vi "Wilt Prototype.vi"() -> ()   [LabVIEW 2009]
uses:
  Globals Wilt.vi
  Dryer.ctl
  Dryer Details.ctl
  Agilent Channel Definition.ctl
panel:
  out "Agilent Channels Array":T1[](array[typedef])
  out "Agilent Station Data Index Array":i32[][](array[numeric])
  out "Agilent Station Data Headers":string[][](array[string])
  in  "GUI Aisle 1A":T2[](array[typedef])=[{"Serial Number"="", "Cycle Count"=0.0, "Station Number"=0, "Dryer Details"={"Station"="", "Cycle Count"="", "Status"="", "Debug ASCII"="", "Note"="", "FILEMNAME"="", "Serial Number"="", "Total Time Drying"=""}, "Sample Record(t, Cycle Count, t-cum,L1, L2, V, Trmb, ASCII, Status) "=[], "Hist Record(Cycle Count, t-comp,L1max, L2max, Tmax) "=[], "Status Color"=0, "Boolean"=FALSE}, {"Serial Number"="", "Cycle Count"=0.0, "Station Number"=0, "Dryer Details"={"Station"="", "Cycle Count"="", "Status"="", "Debug ASCII"="", "Note"="", "FILEMNAME"="", "Serial Number"="", "Total Time Drying"=""}, "Sample Record(t, Cycle Count, t-cum,L1, L2, V, Trmb, ASCII, Status) "=[], "Hist Record(Cycle Count, t-comp,L1max, L2max, Tmax) "=[], "Status Color"=0, "Boolean"=FALSE}, {"Serial Number"="", "Cycle Count"=0.0, "Station Number"=0, "Dryer Details"={"Station"="", "Cycle Count"="", "Status"="", "Debug ASCII"="", "Note"="", "FILEMNAME"="", "Serial Number"="", "Total Time Drying"=""}, "Sample Record(t, Cycle Count, t-cum,L1, L2, V, Trmb, ASCII, Status) "=[], "Hist Record(Cycle Count, t-comp,L1max, L2max, Tmax) "=[], "Status Color"=0, "Boolean"=FALSE}, {"Serial Number"="", "Cycle Count"=0.0, "Station Number"=0, "Dryer Details"={"Station"="", "Cycle Count"="", "Status"="", "Debug ASCII"="", "Note"="", "FILEMNAME"="", "Serial Number"="", "Total Time Drying"=""}, "Sample Record(t, Cycle Count, t-cum,L1, L2, V, Trmb, ASCII, Status) "=[], "Hist Record(Cycle Count, t-comp,L1max, L2max, Tmax) "=[], "Status Color"=0, "Boolean"=FALSE}, {"Serial Number"="", "Cycle Count"=0.0, "Station Number"=0, "Dryer Details"={"Station"="", "Cycle Count"="", "Status"="", "Debug ASCII"="", "Note"="", "FILEMNAME"="", "Serial Number"="", "Total Time Drying"=""}, "Sample Record(t, Cycle Count, t-cum,L1, L2, V, Trmb, ASCII, Status) "=[], "Hist Record(Cycle Count, t-comp,L1max, L2max, Tmax) "=[], "Status Color"=0, "Boolean"=FALSE}, {"Serial Number"="", "Cycle Count"=0.0, "Station Number"=0, "Dryer Details"={"Station"="", "Cycle Count"="", "Status"="", "Debug ASCII"="", "Note"="", "FILEMNAME"="", "Serial Number"="", "Total Time Drying"=""}, "Sample Record(t, Cycle Count, t-cum,L1, L2, V, Trmb, ASCII, Status) "=[], "Hist Record(Cycle Count, t-comp,L1max, L2max, Tmax) "=[], "Status Color"=0, "Boolean"=FALSE}, {"Serial Number"="", "Cycle Count"=0.0, "Station Number"=0, "Dryer Details"={"Station"="", "Cycle Count"="", "Status"="", "Debug ASCII"="", "Note"="", "FILEMNAME"="", "Serial Number"="", "Total Time Drying"=""}, "Sample Record(t, Cycle Count, t-cum,L1, L2, V, Trmb, ASCII, Status) "=[], "Hist Record(Cycle Count, t-comp,L1max, L2max, Tmax) "=[], "Status Color"=0, "Boolean"=FALSE}, {"Serial Number"="", "Cycle Count"=0.0, "Station Number"=0, "Dryer Details"={"Station"="", "Cycle Count"="", "Status"="", "Debug ASCII"="", "Note"="", "FILEMNAME"="", "Serial Number"="", "Total Time Drying"=""}, "Sample Record(t, Cycle Count, t-cum,L1, L2, V, Trmb, ASCII, Status) "=[], "Hist Record(Cycle Count, t-comp,L1max, L2max, Tmax) "=[], "Status Color"=0, "Boolean"=TRUE}] {"Station Number" format="%02.0f"; "Cycle Count" format="%0#4_4g"}
  in  "GUI Aisle 1":T2[](array[typedef])=[{"Serial Number"="", "Cycle Count"=0.0, "Station Number"=0, "Dryer Details"={"Station"="", "Cycle Count"="", "Status"="", "Debug ASCII"="", "Note"="", "FILEMNAME"="", "Serial Number"="", "Total Time Drying"=""}, "Sample Record(t, Cycle Count, t-cum,L1, L2, V, Trmb, ASCII, Status) "=[], "Hist Record(Cycle Count, t-comp,L1max, L2max, Tmax) "=[], "Status Color"=0, "Boolean"=FALSE}, {"Serial Number"="", "Cycle Count"=0.0, "Station Number"=0, "Dryer Details"={"Station"="", "Cycle Count"="", "Status"="", "Debug ASCII"="", "Note"="", "FILEMNAME"="", "Serial Number"="", "Total Time Drying"=""}, "Sample Record(t, Cycle Count, t-cum,L1, L2, V, Trmb, ASCII, Status) "=[], "Hist Record(Cycle Count, t-comp,L1max, L2max, Tmax) "=[], "Status Color"=0, "Boolean"=FALSE}, {"Serial Number"="", "Cycle Count"=0.0, "Station Number"=0, "Dryer Details"={"Station"="", "Cycle Count"="", "Status"="", "Debug ASCII"="", "Note"="", "FILEMNAME"="", "Serial Number"="", "Total Time Drying"=""}, "Sample Record(t, Cycle Count, t-cum,L1, L2, V, Trmb, ASCII, Status) "=[], "Hist Record(Cycle Count, t-comp,L1max, L2max, Tmax) "=[], "Status Color"=0, "Boolean"=FALSE}, {"Serial Number"="", "Cycle Count"=0.0, "Station Number"=0, "Dryer Details"={"Station"="", "Cycle Count"="", "Status"="", "Debug ASCII"="", "Note"="", "FILEMNAME"="", "Serial Number"="", "Total Time Drying"=""}, "Sample Record(t, Cycle Count, t-cum,L1, L2, V, Trmb, ASCII, Status) "=[], "Hist Record(Cycle Count, t-comp,L1max, L2max, Tmax) "=[], "Status Color"=0, "Boolean"=FALSE}, {"Serial Number"="", "Cycle Count"=0.0, "Station Number"=0, "Dryer Details"={"Station"="", "Cycle Count"="", "Status"="", "Debug ASCII"="", "Note"="", "FILEMNAME"="", "Serial Number"="", "Total Time Drying"=""}, "Sample Record(t, Cycle Count, t-cum,L1, L2, V, Trmb, ASCII, Status) "=[], "Hist Record(Cycle Count, t-comp,L1max, L2max, Tmax) "=[], "Status Color"=0, "Boolean"=FALSE}, {"Serial Number"="", "Cycle Count"=0.0, "Station Number"=0, "Dryer Details"={"Station"="", "Cycle Count"="", "Status"="", "Debug ASCII"="", "Note"="", "FILEMNAME"="", "Serial Number"="", "Total Time Drying"=""}, "Sample Record(t, Cycle Count, t-cum,L1, L2, V, Trmb, ASCII, Status) "=[], "Hist Record(Cycle Count, t-comp,L1max, L2max, Tmax) "=[], "Status Color"=0, "Boolean"=FALSE}, {"Serial Number"="", "Cycle Count"=0.0, "Station Number"=0, "Dryer Details"={"Station"="", "Cycle Count"="", "Status"="", "Debug ASCII"="", "Note"="", "FILEMNAME"="", "Serial Number"="", "Total Time Drying"=""}, "Sample Record(t, Cycle Count, t-cum,L1, L2, V, Trmb, ASCII, Status) "=[], "Hist Record(Cycle Count, t-comp,L1max, L2max, Tmax) "=[], "Status Color"=0, "Boolean"=FALSE}, {"Serial Number"="", "Cycle Count"=0.0, "Station Number"=0, "Dryer Details"={"Station"="", "Cycle Count"="", "Status"="", "Debug ASCII"="", "Note"="", "FILEMNAME"="", "Serial Number"="", "Total Time Drying"=""}, "Sample Record(t, Cycle Count, t-cum,L1, L2, V, Trmb, ASCII, Status) "=[], "Hist Record(Cycle Count, t-comp,L1max, L2max, Tmax) "=[], "Status Color"=0, "Boolean"=FALSE}, {"Serial Number"="", "Cycle Count"=0.0, "Station Number"=0, "Dryer Details"={"Station"="", "Cycle Count"="", "Status"="", "Debug ASCII"="", "Note"="", "FILEMNAME"="", "Serial Number"="", "Total Time Drying"=""}, "Sample Record(t, Cycle Count, t-cum,L1, L2, V, Trmb, ASCII, Status) "=[], "Hist Record(Cycle Count, t-comp,L1max, L2max, Tmax) "=[], "Status Color"=0, "Boolean"=FALSE}, {"Serial Number"="", "Cycle Count"=0.0, "Station Number"=0, "Dryer Details"={"Station"="", "Cycle Count"="", "Status"="", "Debug ASCII"="", "Note"="", "FILEMNAME"="", "Serial Number"="", "Total Time Drying"=""}, "Sample Record(t, Cycle Count, t-cum,L1, L2, V, Trmb, ASCII, Status) "=[], "Hist Record(Cycle Count, t-comp,L1max, L2max, Tmax) "=[], "Status Color"=0, "Boolean"=FALSE}, {"Serial Number"="", "Cycle Count"=0.0, "Station Number"=0, "Dryer Details"={"Station"="", "Cycle Count"="", "Status"="", "Debug ASCII"="", "Note"="", "FILEMNAME"="", "Serial Number"="", "Total Time Drying"=""}, "Sample Record(t, Cycle Count, t-cum,L1, L2, V, Trmb, ASCII, Status) "=[], "Hist Record(Cycle Count, t-comp,L1max, L2max, Tmax) "=[], "Status Color"=0, "Boolean"=FALSE}, {"Serial Number"="", "Cycle Count"=0.0, "Station Number"=0, "Dryer Details"={"Station"="", "Cycle Count"="", "Status"="", "Debug ASCII"="", "Note"="", "FILEMNAME"="", "Serial Number"="", "Total Time Drying"=""}, "Sample Record(t, Cycle Count, t-cum,L1, L2, V, Trmb, ASCII, Status) "=[], "Hist Record(Cycle Count, t-comp,L1max, L2max, Tmax) "=[], "Status Color"=0, "Boolean"=TRUE}] {"Station Number" format="%02.0f"; "Cycle Count" format="%0#4_4g"}
  in  "GUI Aisle 2":T2[](array[typedef])=[{"Serial Number"="", "Cycle Count"=0.0, "Station Number"=0, "Dryer Details"={"Station"="", "Cycle Count"="", "Status"="", "Debug ASCII"="", "Note"="", "FILEMNAME"="", "Serial Number"="", "Total Time Drying"=""}, "Sample Record(t, Cycle Count, t-cum,L1, L2, V, Trmb, ASCII, Status) "=[], "Hist Record(Cycle Count, t-comp,L1max, L2max, Tmax) "=[], "Status Color"=0, "Boolean"=FALSE}, {"Serial Number"="", "Cycle Count"=0.0, "Station Number"=0, "Dryer Details"={"Station"="", "Cycle Count"="", "Status"="", "Debug ASCII"="", "Note"="", "FILEMNAME"="", "Serial Number"="", "Total Time Drying"=""}, "Sample Record(t, Cycle Count, t-cum,L1, L2, V, Trmb, ASCII, Status) "=[], "Hist Record(Cycle Count, t-comp,L1max, L2max, Tmax) "=[], "Status Color"=0, "Boolean"=FALSE}, {"Serial Number"="", "Cycle Count"=0.0, "Station Number"=0, "Dryer Details"={"Station"="", "Cycle Count"="", "Status"="", "Debug ASCII"="", "Note"="", "FILEMNAME"="", "Serial Number"="", "Total Time Drying"=""}, "Sample Record(t, Cycle Count, t-cum,L1, L2, V, Trmb, ASCII, Status) "=[], "Hist Record(Cycle Count, t-comp,L1max, L2max, Tmax) "=[], "Status Color"=0, "Boolean"=FALSE}, {"Serial Number"="", "Cycle Count"=0.0, "Station Number"=0, "Dryer Details"={"Station"="", "Cycle Count"="", "Status"="", "Debug ASCII"="", "Note"="", "FILEMNAME"="", "Serial Number"="", "Total Time Drying"=""}, "Sample Record(t, Cycle Count, t-cum,L1, L2, V, Trmb, ASCII, Status) "=[], "Hist Record(Cycle Count, t-comp,L1max, L2max, Tmax) "=[], "Status Color"=0, "Boolean"=FALSE}, {"Serial Number"="", "Cycle Count"=0.0, "Station Number"=0, "Dryer Details"={"Station"="", "Cycle Count"="", "Status"="", "Debug ASCII"="", "Note"="", "FILEMNAME"="", "Serial Number"="", "Total Time Drying"=""}, "Sample Record(t, Cycle Count, t-cum,L1, L2, V, Trmb, ASCII, Status) "=[], "Hist Record(Cycle Count, t-comp,L1max, L2max, Tmax) "=[], "Status Color"=0, "Boolean"=FALSE}, {"Serial Number"="", "Cycle Count"=0.0, "Station Number"=0, "Dryer Details"={"Station"="", "Cycle Count"="", "Status"="", "Debug ASCII"="", "Note"="", "FILEMNAME"="", "Serial Number"="", "Total Time Drying"=""}, "Sample Record(t, Cycle Count, t-cum,L1, L2, V, Trmb, ASCII, Status) "=[], "Hist Record(Cycle Count, t-comp,L1max, L2max, Tmax) "=[], "Status Color"=0, "Boolean"=FALSE}, {"Serial Number"="", "Cycle Count"=0.0, "Station Number"=0, "Dryer Details"={"Station"="", "Cycle Count"="", "Status"="", "Debug ASCII"="", "Note"="", "FILEMNAME"="", "Serial Number"="", "Total Time Drying"=""}, "Sample Record(t, Cycle Count, t-cum,L1, L2, V, Trmb, ASCII, Status) "=[], "Hist Record(Cycle Count, t-comp,L1max, L2max, Tmax) "=[], "Status Color"=0, "Boolean"=FALSE}, {"Serial Number"="", "Cycle Count"=0.0, "Station Number"=0, "Dryer Details"={"Station"="", "Cycle Count"="", "Status"="", "Debug ASCII"="", "Note"="", "FILEMNAME"="", "Serial Number"="", "Total Time Drying"=""}, "Sample Record(t, Cycle Count, t-cum,L1, L2, V, Trmb, ASCII, Status) "=[], "Hist Record(Cycle Count, t-comp,L1max, L2max, Tmax) "=[], "Status Color"=0, "Boolean"=FALSE}, {"Serial Number"="", "Cycle Count"=0.0, "Station Number"=0, "Dryer Details"={"Station"="", "Cycle Count"="", "Status"="", "Debug ASCII"="", "Note"="", "FILEMNAME"="", "Serial Number"="", "Total Time Drying"=""}, "Sample Record(t, Cycle Count, t-cum,L1, L2, V, Trmb, ASCII, Status) "=[], "Hist Record(Cycle Count, t-comp,L1max, L2max, Tmax) "=[], "Status Color"=0, "Boolean"=FALSE}, {"Serial Number"="", "Cycle Count"=0.0, "Station Number"=0, "Dryer Details"={"Station"="", "Cycle Count"="", "Status"="", "Debug ASCII"="", "Note"="", "FILEMNAME"="", "Serial Number"="", "Total Time Drying"=""}, "Sample Record(t, Cycle Count, t-cum,L1, L2, V, Trmb, ASCII, Status) "=[], "Hist Record(Cycle Count, t-comp,L1max, L2max, Tmax) "=[], "Status Color"=0, "Boolean"=FALSE}, {"Serial Number"="", "Cycle Count"=0.0, "Station Number"=0, "Dryer Details"={"Station"="", "Cycle Count"="", "Status"="", "Debug ASCII"="", "Note"="", "FILEMNAME"="", "Serial Number"="", "Total Time Drying"=""}, "Sample Record(t, Cycle Count, t-cum,L1, L2, V, Trmb, ASCII, Status) "=[], "Hist Record(Cycle Count, t-comp,L1max, L2max, Tmax) "=[], "Status Color"=0, "Boolean"=FALSE}, {"Serial Number"="", "Cycle Count"=0.0, "Station Number"=0, "Dryer Details"={"Station"="", "Cycle Count"="", "Status"="", "Debug ASCII"="", "Note"="", "FILEMNAME"="", "Serial Number"="", "Total Time Drying"=""}, "Sample Record(t, Cycle Count, t-cum,L1, L2, V, Trmb, ASCII, Status) "=[], "Hist Record(Cycle Count, t-comp,L1max, L2max, Tmax) "=[], "Status Color"=0, "Boolean"=TRUE}] {"Station Number" format="%02.0f"; "Cycle Count" format="%0#4_4g"}
  in  "GUI Aisle 3":T2[](array[typedef])=[{"Serial Number"="", "Cycle Count"=0.0, "Station Number"=0, "Dryer Details"={"Station"="", "Cycle Count"="", "Status"="", "Debug ASCII"="", "Note"="", "FILEMNAME"="", "Serial Number"="", "Total Time Drying"=""}, "Sample Record(t, Cycle Count, t-cum,L1, L2, V, Trmb, ASCII, Status) "=[], "Hist Record(Cycle Count, t-comp,L1max, L2max, Tmax) "=[], "Status Color"=0, "Boolean"=FALSE}, {"Serial Number"="", "Cycle Count"=0.0, "Station Number"=0, "Dryer Details"={"Station"="", "Cycle Count"="", "Status"="", "Debug ASCII"="", "Note"="", "FILEMNAME"="", "Serial Number"="", "Total Time Drying"=""}, "Sample Record(t, Cycle Count, t-cum,L1, L2, V, Trmb, ASCII, Status) "=[], "Hist Record(Cycle Count, t-comp,L1max, L2max, Tmax) "=[], "Status Color"=0, "Boolean"=FALSE}, {"Serial Number"="", "Cycle Count"=0.0, "Station Number"=0, "Dryer Details"={"Station"="", "Cycle Count"="", "Status"="", "Debug ASCII"="", "Note"="", "FILEMNAME"="", "Serial Number"="", "Total Time Drying"=""}, "Sample Record(t, Cycle Count, t-cum,L1, L2, V, Trmb, ASCII, Status) "=[], "Hist Record(Cycle Count, t-comp,L1max, L2max, Tmax) "=[], "Status Color"=0, "Boolean"=FALSE}, {"Serial Number"="", "Cycle Count"=0.0, "Station Number"=0, "Dryer Details"={"Station"="", "Cycle Count"="", "Status"="", "Debug ASCII"="", "Note"="", "FILEMNAME"="", "Serial Number"="", "Total Time Drying"=""}, "Sample Record(t, Cycle Count, t-cum,L1, L2, V, Trmb, ASCII, Status) "=[], "Hist Record(Cycle Count, t-comp,L1max, L2max, Tmax) "=[], "Status Color"=0, "Boolean"=FALSE}, {"Serial Number"="", "Cycle Count"=0.0, "Station Number"=0, "Dryer Details"={"Station"="", "Cycle Count"="", "Status"="", "Debug ASCII"="", "Note"="", "FILEMNAME"="", "Serial Number"="", "Total Time Drying"=""}, "Sample Record(t, Cycle Count, t-cum,L1, L2, V, Trmb, ASCII, Status) "=[], "Hist Record(Cycle Count, t-comp,L1max, L2max, Tmax) "=[], "Status Color"=0, "Boolean"=FALSE}, {"Serial Number"="", "Cycle Count"=0.0, "Station Number"=0, "Dryer Details"={"Station"="", "Cycle Count"="", "Status"="", "Debug ASCII"="", "Note"="", "FILEMNAME"="", "Serial Number"="", "Total Time Drying"=""}, "Sample Record(t, Cycle Count, t-cum,L1, L2, V, Trmb, ASCII, Status) "=[], "Hist Record(Cycle Count, t-comp,L1max, L2max, Tmax) "=[], "Status Color"=0, "Boolean"=FALSE}, {"Serial Number"="", "Cycle Count"=0.0, "Station Number"=0, "Dryer Details"={"Station"="", "Cycle Count"="", "Status"="", "Debug ASCII"="", "Note"="", "FILEMNAME"="", "Serial Number"="", "Total Time Drying"=""}, "Sample Record(t, Cycle Count, t-cum,L1, L2, V, Trmb, ASCII, Status) "=[], "Hist Record(Cycle Count, t-comp,L1max, L2max, Tmax) "=[], "Status Color"=0, "Boolean"=FALSE}, {"Serial Number"="", "Cycle Count"=0.0, "Station Number"=0, "Dryer Details"={"Station"="", "Cycle Count"="", "Status"="", "Debug ASCII"="", "Note"="", "FILEMNAME"="", "Serial Number"="", "Total Time Drying"=""}, "Sample Record(t, Cycle Count, t-cum,L1, L2, V, Trmb, ASCII, Status) "=[], "Hist Record(Cycle Count, t-comp,L1max, L2max, Tmax) "=[], "Status Color"=0, "Boolean"=FALSE}, {"Serial Number"="", "Cycle Count"=0.0, "Station Number"=0, "Dryer Details"={"Station"="", "Cycle Count"="", "Status"="", "Debug ASCII"="", "Note"="", "FILEMNAME"="", "Serial Number"="", "Total Time Drying"=""}, "Sample Record(t, Cycle Count, t-cum,L1, L2, V, Trmb, ASCII, Status) "=[], "Hist Record(Cycle Count, t-comp,L1max, L2max, Tmax) "=[], "Status Color"=0, "Boolean"=FALSE}, {"Serial Number"="", "Cycle Count"=0.0, "Station Number"=0, "Dryer Details"={"Station"="", "Cycle Count"="", "Status"="", "Debug ASCII"="", "Note"="", "FILEMNAME"="", "Serial Number"="", "Total Time Drying"=""}, "Sample Record(t, Cycle Count, t-cum,L1, L2, V, Trmb, ASCII, Status) "=[], "Hist Record(Cycle Count, t-comp,L1max, L2max, Tmax) "=[], "Status Color"=0, "Boolean"=FALSE}, {"Serial Number"="", "Cycle Count"=0.0, "Station Number"=0, "Dryer Details"={"Station"="", "Cycle Count"="", "Status"="", "Debug ASCII"="", "Note"="", "FILEMNAME"="", "Serial Number"="", "Total Time Drying"=""}, "Sample Record(t, Cycle Count, t-cum,L1, L2, V, Trmb, ASCII, Status) "=[], "Hist Record(Cycle Count, t-comp,L1max, L2max, Tmax) "=[], "Status Color"=0, "Boolean"=FALSE}, {"Serial Number"="", "Cycle Count"=0.0, "Station Number"=0, "Dryer Details"={"Station"="", "Cycle Count"="", "Status"="", "Debug ASCII"="", "Note"="", "FILEMNAME"="", "Serial Number"="", "Total Time Drying"=""}, "Sample Record(t, Cycle Count, t-cum,L1, L2, V, Trmb, ASCII, Status) "=[], "Hist Record(Cycle Count, t-comp,L1max, L2max, Tmax) "=[], "Status Color"=0, "Boolean"=TRUE}] {"Station Number" format="%02.0f"; "Cycle Count" format="%0#4_4g"}
  in  "GUI Aisle 4":T2[](array[typedef])=[{"Serial Number"="", "Cycle Count"=0.0, "Station Number"=0, "Dryer Details"={"Station"="", "Cycle Count"="", "Status"="", "Debug ASCII"="", "Note"="", "FILEMNAME"="", "Serial Number"="", "Total Time Drying"=""}, "Sample Record(t, Cycle Count, t-cum,L1, L2, V, Trmb, ASCII, Status) "=[], "Hist Record(Cycle Count, t-comp,L1max, L2max, Tmax) "=[], "Status Color"=0, "Boolean"=FALSE}, {"Serial Number"="", "Cycle Count"=0.0, "Station Number"=0, "Dryer Details"={"Station"="", "Cycle Count"="", "Status"="", "Debug ASCII"="", "Note"="", "FILEMNAME"="", "Serial Number"="", "Total Time Drying"=""}, "Sample Record(t, Cycle Count, t-cum,L1, L2, V, Trmb, ASCII, Status) "=[], "Hist Record(Cycle Count, t-comp,L1max, L2max, Tmax) "=[], "Status Color"=0, "Boolean"=FALSE}, {"Serial Number"="", "Cycle Count"=0.0, "Station Number"=0, "Dryer Details"={"Station"="", "Cycle Count"="", "Status"="", "Debug ASCII"="", "Note"="", "FILEMNAME"="", "Serial Number"="", "Total Time Drying"=""}, "Sample Record(t, Cycle Count, t-cum,L1, L2, V, Trmb, ASCII, Status) "=[], "Hist Record(Cycle Count, t-comp,L1max, L2max, Tmax) "=[], "Status Color"=0, "Boolean"=FALSE}, {"Serial Number"="", "Cycle Count"=0.0, "Station Number"=0, "Dryer Details"={"Station"="", "Cycle Count"="", "Status"="", "Debug ASCII"="", "Note"="", "FILEMNAME"="", "Serial Number"="", "Total Time Drying"=""}, "Sample Record(t, Cycle Count, t-cum,L1, L2, V, Trmb, ASCII, Status) "=[], "Hist Record(Cycle Count, t-comp,L1max, L2max, Tmax) "=[], "Status Color"=0, "Boolean"=FALSE}, {"Serial Number"="", "Cycle Count"=0.0, "Station Number"=0, "Dryer Details"={"Station"="", "Cycle Count"="", "Status"="", "Debug ASCII"="", "Note"="", "FILEMNAME"="", "Serial Number"="", "Total Time Drying"=""}, "Sample Record(t, Cycle Count, t-cum,L1, L2, V, Trmb, ASCII, Status) "=[], "Hist Record(Cycle Count, t-comp,L1max, L2max, Tmax) "=[], "Status Color"=0, "Boolean"=FALSE}, {"Serial Number"="", "Cycle Count"=0.0, "Station Number"=0, "Dryer Details"={"Station"="", "Cycle Count"="", "Status"="", "Debug ASCII"="", "Note"="", "FILEMNAME"="", "Serial Number"="", "Total Time Drying"=""}, "Sample Record(t, Cycle Count, t-cum,L1, L2, V, Trmb, ASCII, Status) "=[], "Hist Record(Cycle Count, t-comp,L1max, L2max, Tmax) "=[], "Status Color"=0, "Boolean"=FALSE}, {"Serial Number"="", "Cycle Count"=0.0, "Station Number"=0, "Dryer Details"={"Station"="", "Cycle Count"="", "Status"="", "Debug ASCII"="", "Note"="", "FILEMNAME"="", "Serial Number"="", "Total Time Drying"=""}, "Sample Record(t, Cycle Count, t-cum,L1, L2, V, Trmb, ASCII, Status) "=[], "Hist Record(Cycle Count, t-comp,L1max, L2max, Tmax) "=[], "Status Color"=0, "Boolean"=FALSE}, {"Serial Number"="", "Cycle Count"=0.0, "Station Number"=0, "Dryer Details"={"Station"="", "Cycle Count"="", "Status"="", "Debug ASCII"="", "Note"="", "FILEMNAME"="", "Serial Number"="", "Total Time Drying"=""}, "Sample Record(t, Cycle Count, t-cum,L1, L2, V, Trmb, ASCII, Status) "=[], "Hist Record(Cycle Count, t-comp,L1max, L2max, Tmax) "=[], "Status Color"=0, "Boolean"=FALSE}, {"Serial Number"="", "Cycle Count"=0.0, "Station Number"=0, "Dryer Details"={"Station"="", "Cycle Count"="", "Status"="", "Debug ASCII"="", "Note"="", "FILEMNAME"="", "Serial Number"="", "Total Time Drying"=""}, "Sample Record(t, Cycle Count, t-cum,L1, L2, V, Trmb, ASCII, Status) "=[], "Hist Record(Cycle Count, t-comp,L1max, L2max, Tmax) "=[], "Status Color"=0, "Boolean"=FALSE}, {"Serial Number"="", "Cycle Count"=0.0, "Station Number"=0, "Dryer Details"={"Station"="", "Cycle Count"="", "Status"="", "Debug ASCII"="", "Note"="", "FILEMNAME"="", "Serial Number"="", "Total Time Drying"=""}, "Sample Record(t, Cycle Count, t-cum,L1, L2, V, Trmb, ASCII, Status) "=[], "Hist Record(Cycle Count, t-comp,L1max, L2max, Tmax) "=[], "Status Color"=0, "Boolean"=FALSE}, {"Serial Number"="", "Cycle Count"=0.0, "Station Number"=0, "Dryer Details"={"Station"="", "Cycle Count"="", "Status"="", "Debug ASCII"="", "Note"="", "FILEMNAME"="", "Serial Number"="", "Total Time Drying"=""}, "Sample Record(t, Cycle Count, t-cum,L1, L2, V, Trmb, ASCII, Status) "=[], "Hist Record(Cycle Count, t-comp,L1max, L2max, Tmax) "=[], "Status Color"=0, "Boolean"=FALSE}, {"Serial Number"="", "Cycle Count"=0.0, "Station Number"=0, "Dryer Details"={"Station"="", "Cycle Count"="", "Status"="", "Debug ASCII"="", "Note"="", "FILEMNAME"="", "Serial Number"="", "Total Time Drying"=""}, "Sample Record(t, Cycle Count, t-cum,L1, L2, V, Trmb, ASCII, Status) "=[], "Hist Record(Cycle Count, t-comp,L1max, L2max, Tmax) "=[], "Status Color"=0, "Boolean"=TRUE}] {"Station Number" format="%02.0f"; "Cycle Count" format="%0#4_4g"}
  out "Elapsed Time (sec)":dbl format="%.2f"
  in  "Tab Control":enum32{"Config Variables", "Page 2", "Page 3"}(tab)
  in  "DAQ Delay":i32=1000
  out "All Com Array":i32[](array[numeric])=[100, 2, 3, 4, 5, 6, 7, 8, 9, 10, 11, 12, 13, 14, 15, 16, 17, 18, 19, 20, 21, 22, 23, 24, 25, 26, 27, 28, 29, 30, 31, 32, 33, 34, 35, 36, 37, 38, 39, 40, 41, 42, 43, 44, 45, 46, 47, 48, 49, 50, 51, 52, 53, 54, 55, 56]
  out "Init Complete":bool=TRUE
  out "Test Complete":bool
  in  "Simulation":bool
  in  "Data File Directory":path
  in  "Dryer To Save":T2 {"Station Number" format="%02.0f"; "Cycle Count" format="%0#4_4g"}
  out "Current Serial Output Array":string[](array[string])
  out "Agilent Refs":refnum<visa-resource-name>[](array[refnum])=["AGILENT1", "AGILENT2", "AGILENT3", "AGILENT4", "AGILENT5"]
  out "Agilent Refs Var":refnum<visa-resource-name>[](array[refnum])=["AGILENT1", "AGILENT2", "AGILENT3", "AGILENT4", "AGILENT5"]
  out "Current Agilent Data":dbl[][](array[numeric])
  out "Gathering Data Latch":bool=TRUE
  out "Current Status Array":cluster{"Color":u32, "Status":string}[](array[cluster])
  in  "Stop Test":bool
  in  "Fault":u32(colorbox)=16711680
  in  "Stopped":u32(colorbox)=16776960
  in  "Running":u32(colorbox)=6618880
  in  "No Com":u32(colorbox)
  # "WILT DRYER Test"
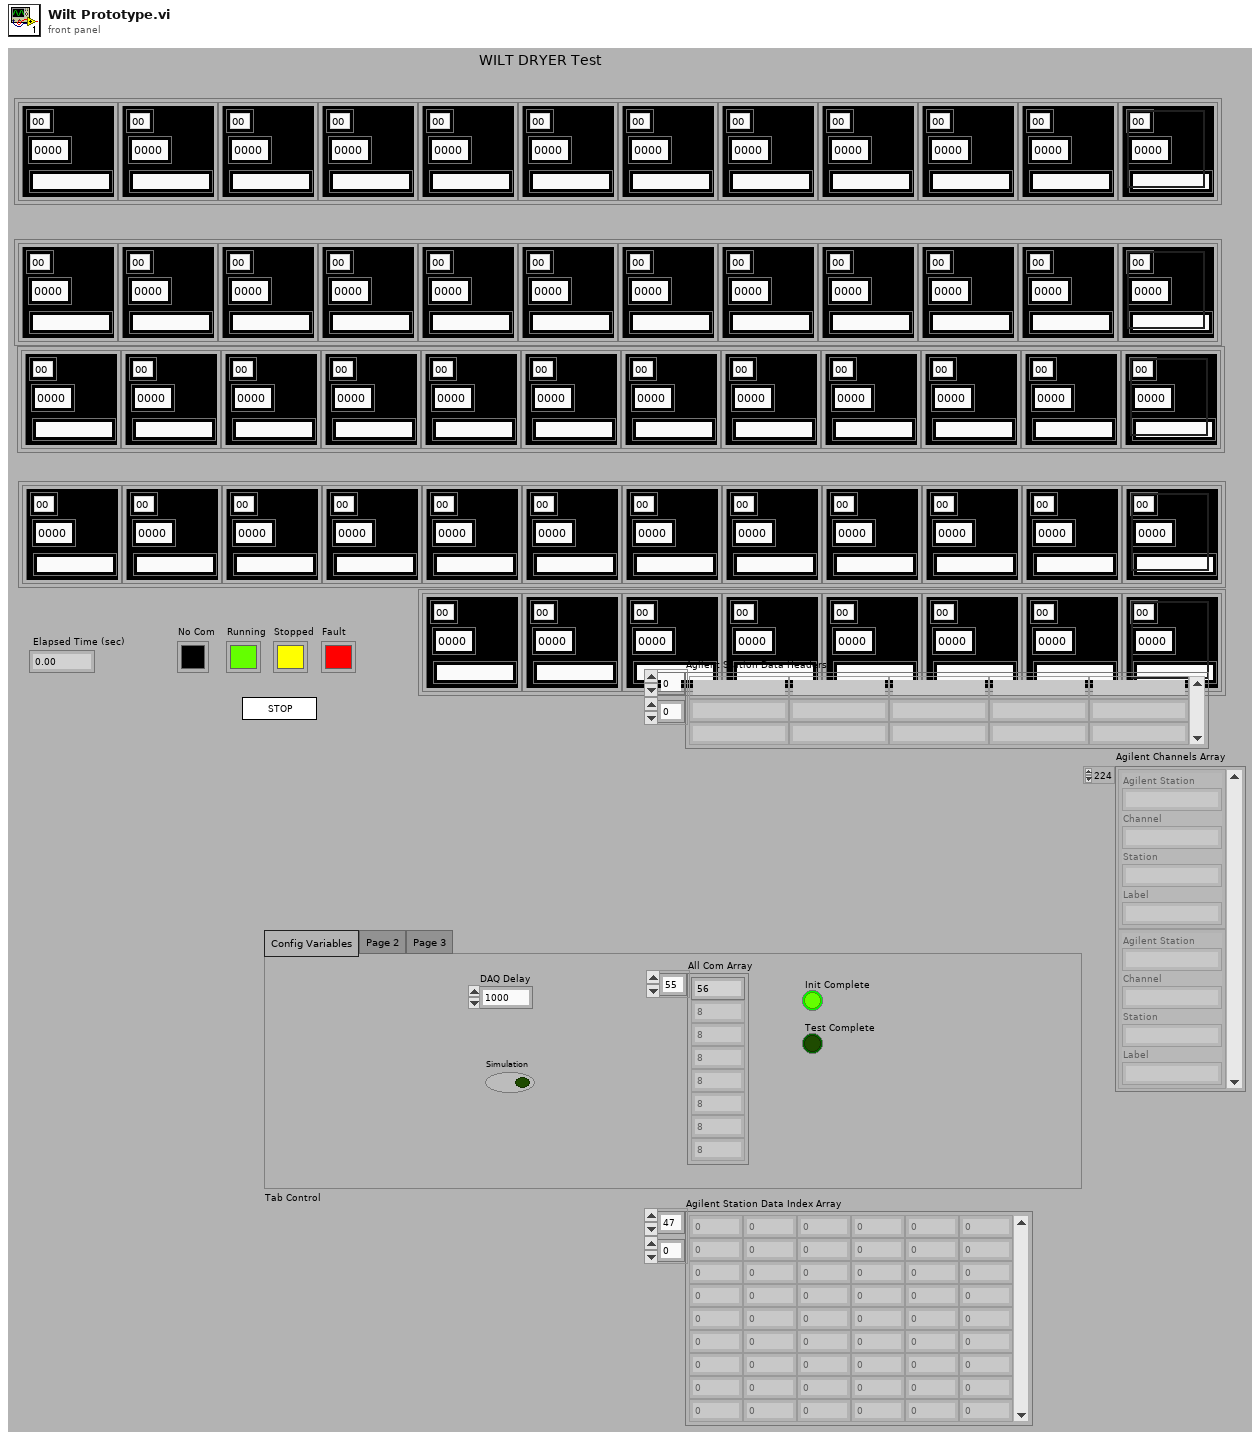
[diagram p1: front panel]
types:
  T1 = typedef "Agilent Channel Definition.ctl" = cluster{"Channel":string, "Station":string, "Label":string, "Agilent Station":string}
  T2 = typedef "Dryer.ctl" = cluster{"Serial Number":string, "Cycle Count":dbl, "Station Number":u8, "Dryer Details":T3, "Sample Record(t, Cycle Count, t-cum,L1, L2, V, Trmb, ASCII, Status) ":string[][], "Hist Record(Cycle Count, t-comp,L1max, L2max, Tmax) ":string[][], "Status Color":u32, "Boolean":bool}
  T3 = typedef "Dryer Details.ctl" = cluster{"Station":string, "Cycle Count":string, "Status":string, "Debug ASCII":string, "Note":string, "FILEMNAME":string, "Serial Number":string, "Total Time Drying":string}
  T4 = enum32{"invalid app kind", "Development System", "Run Time System", "Student Edition", "Embedded LabVIEW", "Evaluation", "Custom"}
  T5 = enum16{"Init Station Number", "Update Detail Data", "Update Status"}
  T6 = enum32{"Invalid", "Standard", "Closed", "Hidden", "Minimized", "Maximized"}
  T7 = cluster{"Core":cluster{"Current VI Reference":refnum<vi>, "Close Panel on Exit?":bool}, "UI Refs":refnum<vi>[], "Agilent Refs":refnum<visa-resource-name>[], "GUI Aisle 4":T2[], "GUI Aisle 3":T2[], "GUI Aisle 2":T2[], "GUI Aisle 1A":T2[], "GUI Aisle 1":T2[]}
  T8 = cluster{"Current VI Reference":refnum<vi>, "Close Panel on Exit?":bool}
  T9 = enum16{"Init Com Port", "SendCMD", "ReadPort", "Close Port", "Simulate Diag Data", "Simulate Dryer"}
  T10 = cluster{"GUI Aisle 1":T2[], "GUI Aisle 1A":T2[], "GUI Aisle 2":T2[], "GUI Aisle 3":T2[], "GUI Aisle 4":T2[], "Dryer To Save":T2}
  T11 = cluster{"Agilent Refs Var":refnum<visa-resource-name>[], "All Com Array":i32[], "Elapsed Time (sec)":dbl}
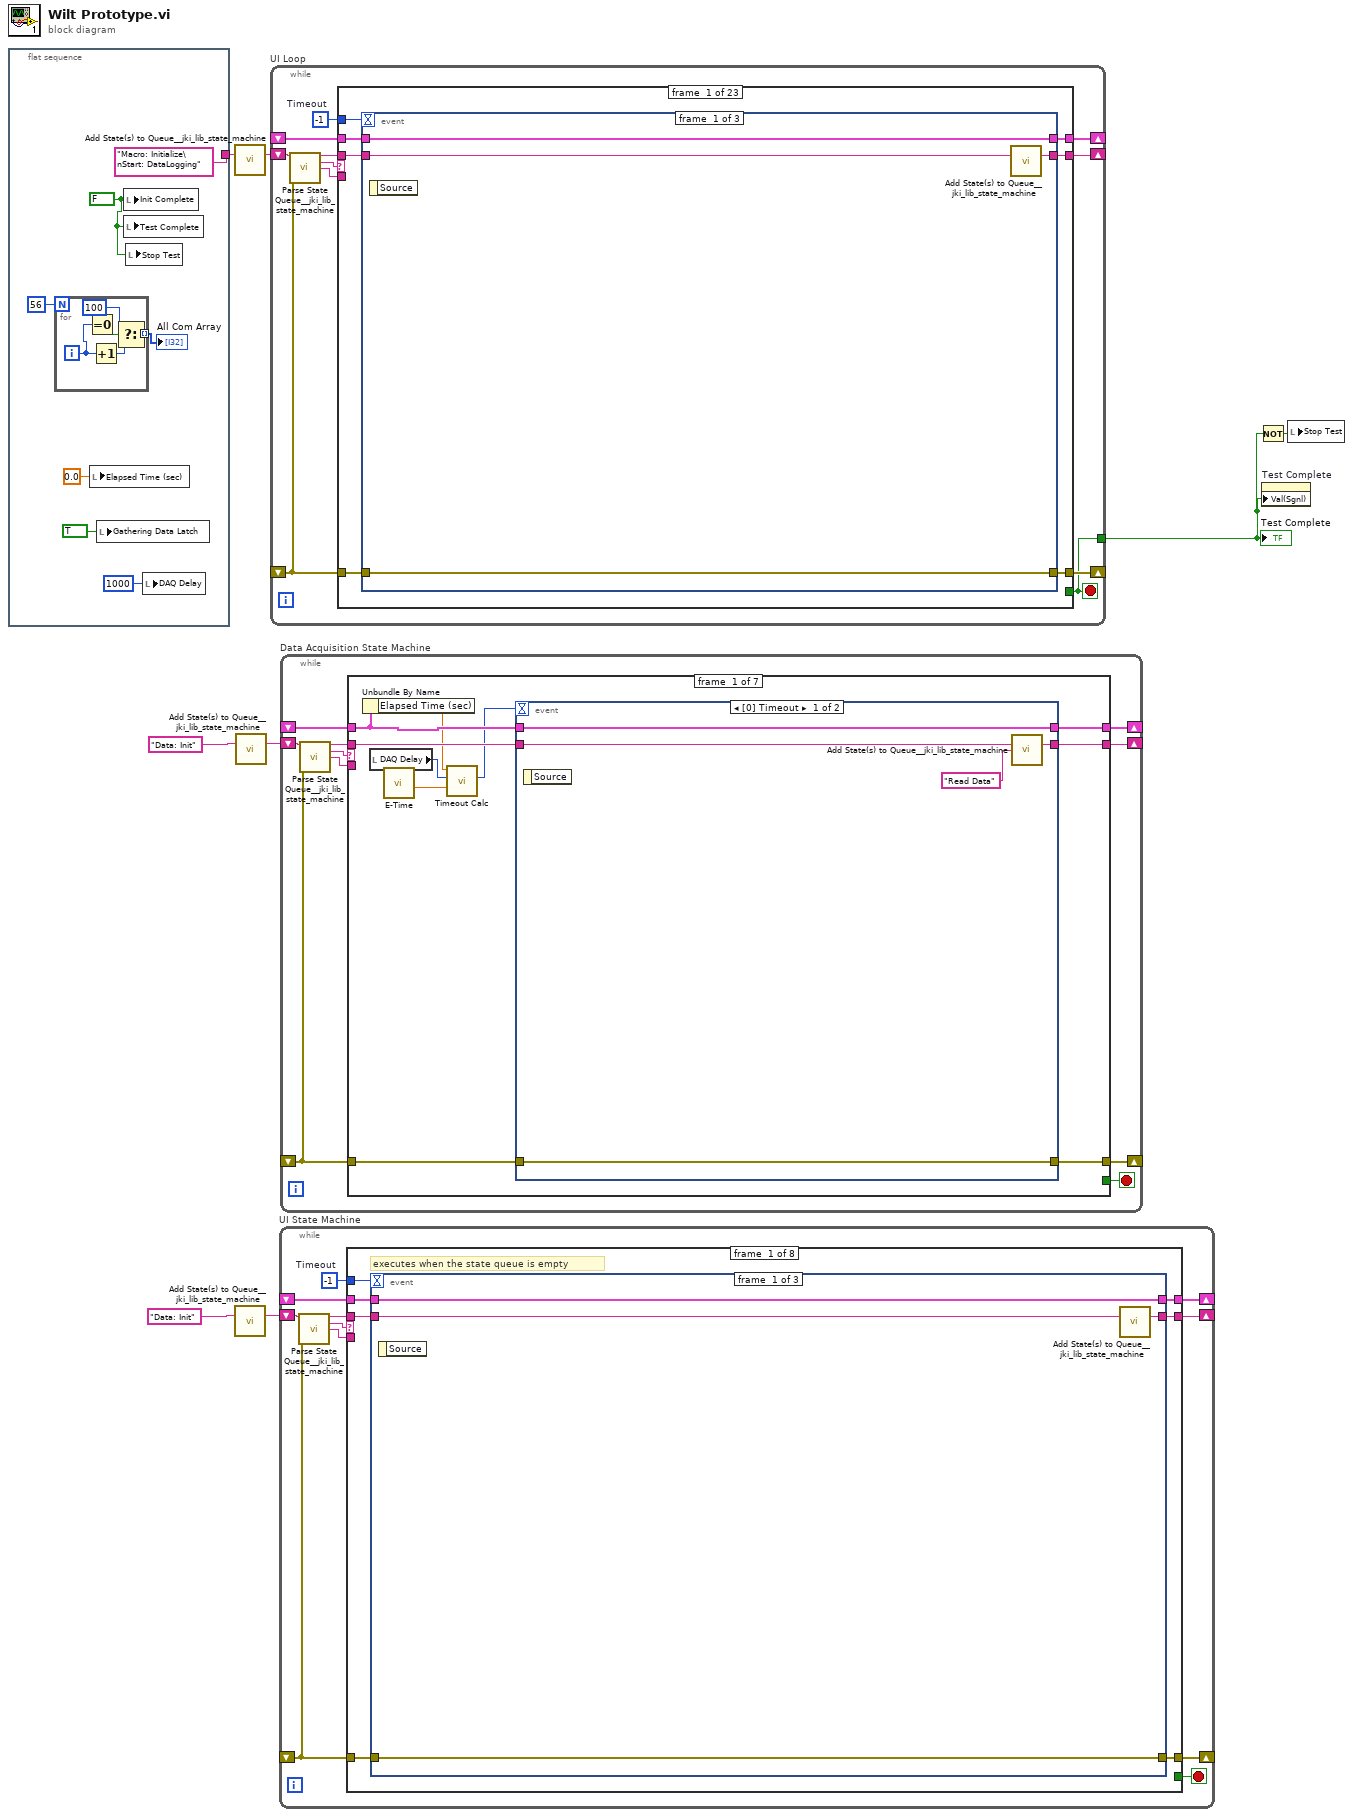
[diagram p0: block diagram]
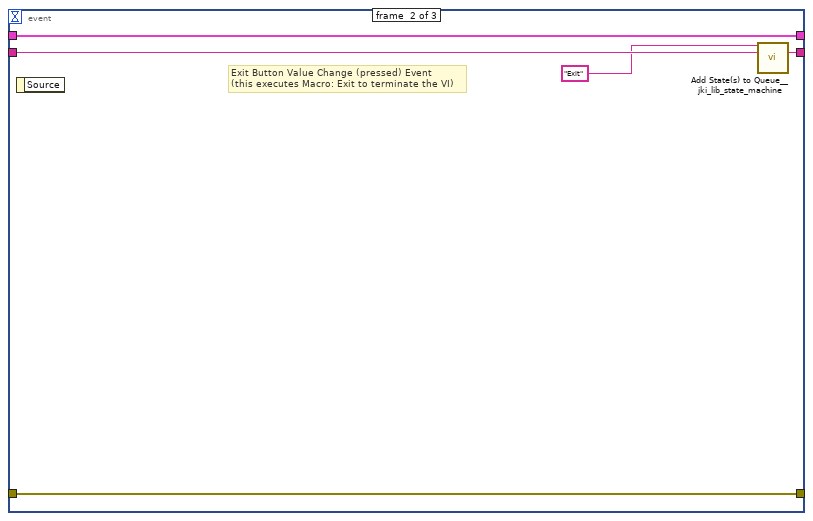
[diagram p2: hidden frame]
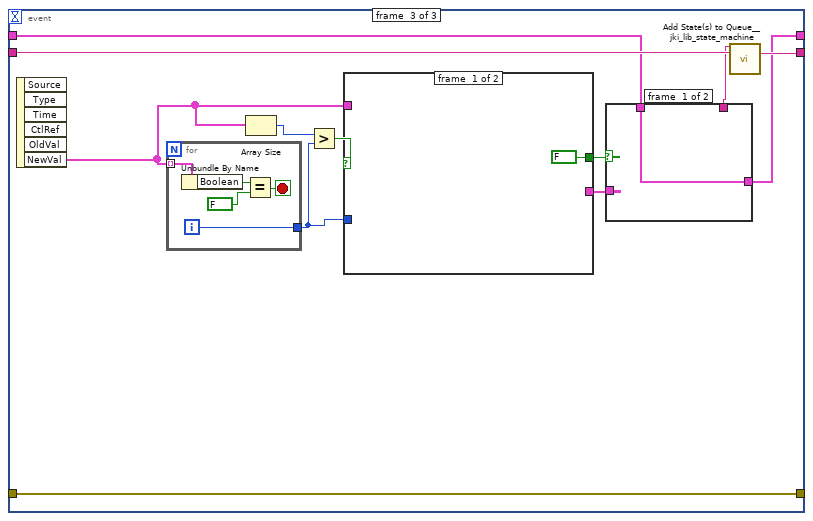
[diagram p3: hidden frame]
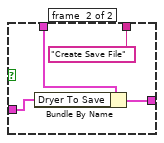
[diagram p4: hidden frame]
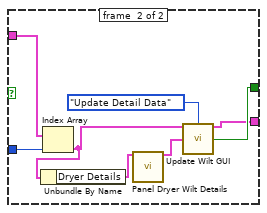
[diagram p5: hidden frame]
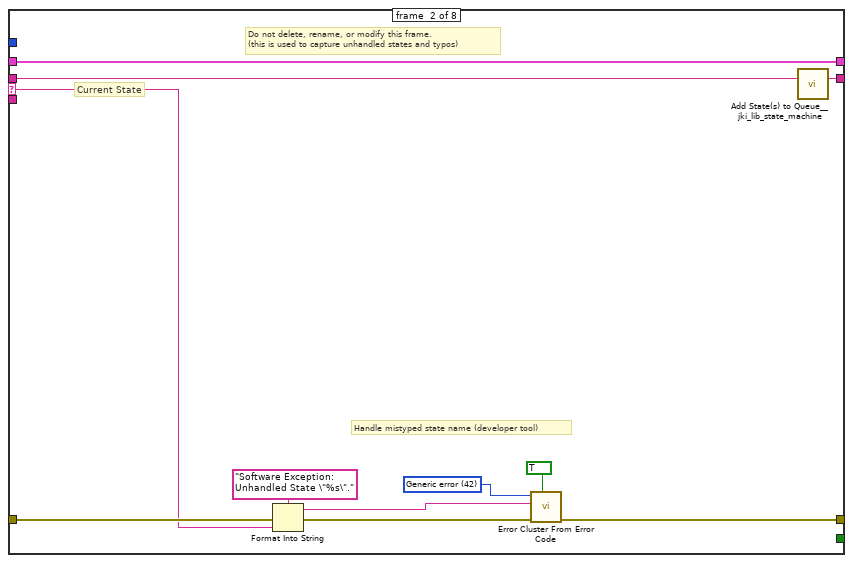
[diagram p6: hidden frame]
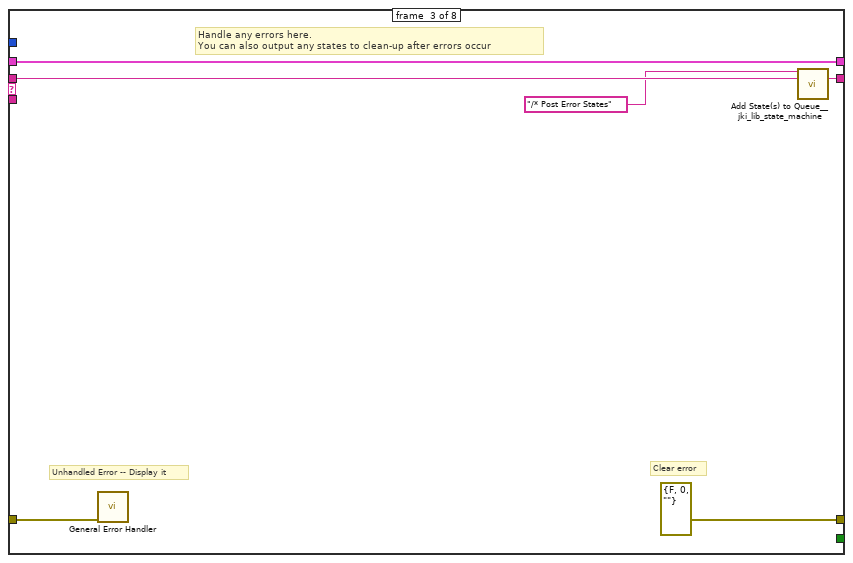
[diagram p7: hidden frame]
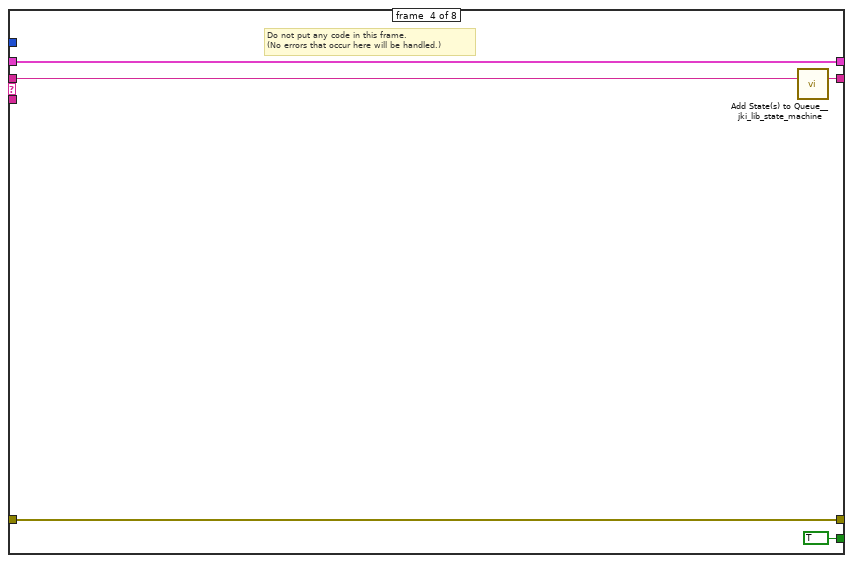
[diagram p8: hidden frame]
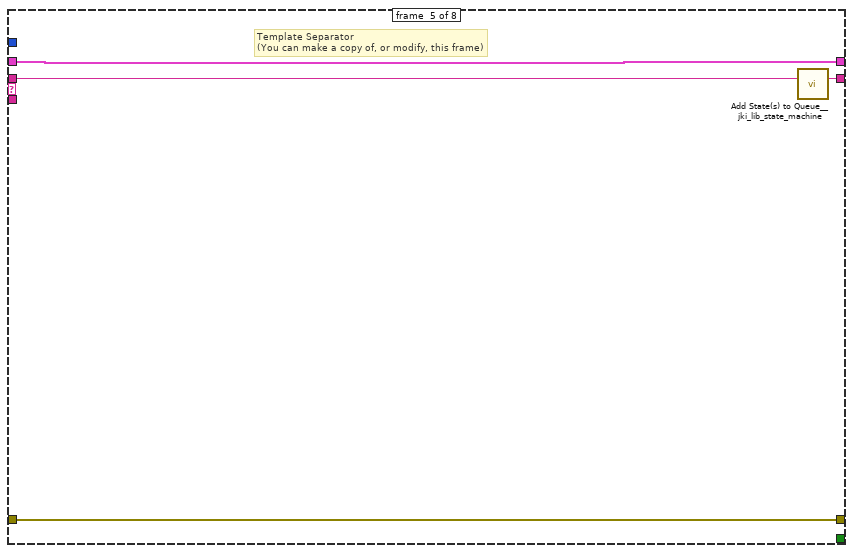
[diagram p9: hidden frame]
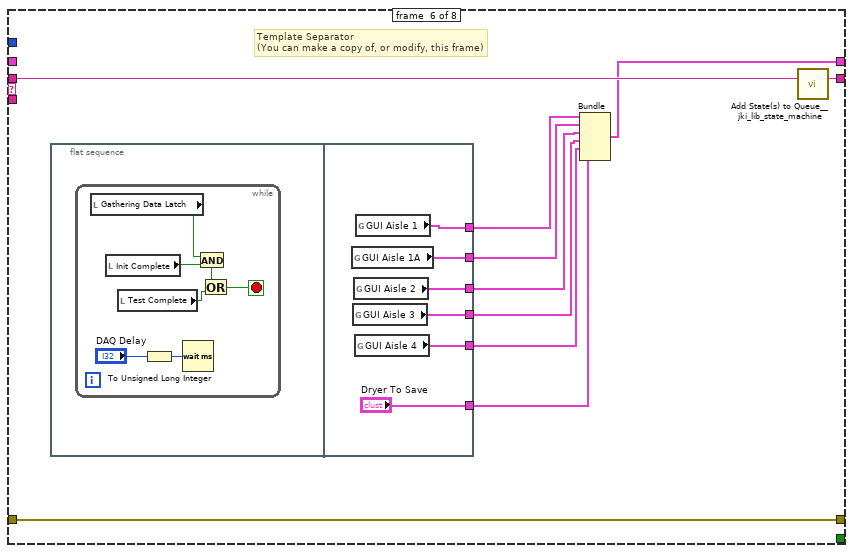
[diagram p10: hidden frame]
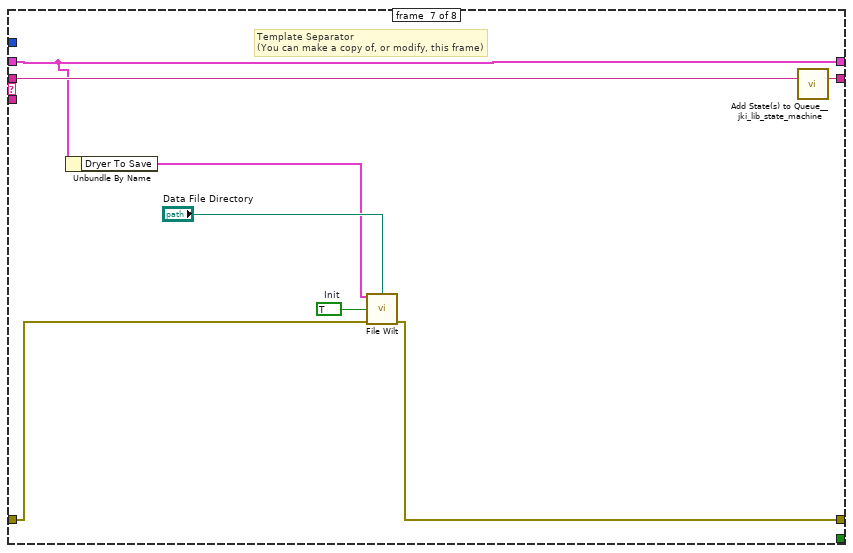
[diagram p11: hidden frame]
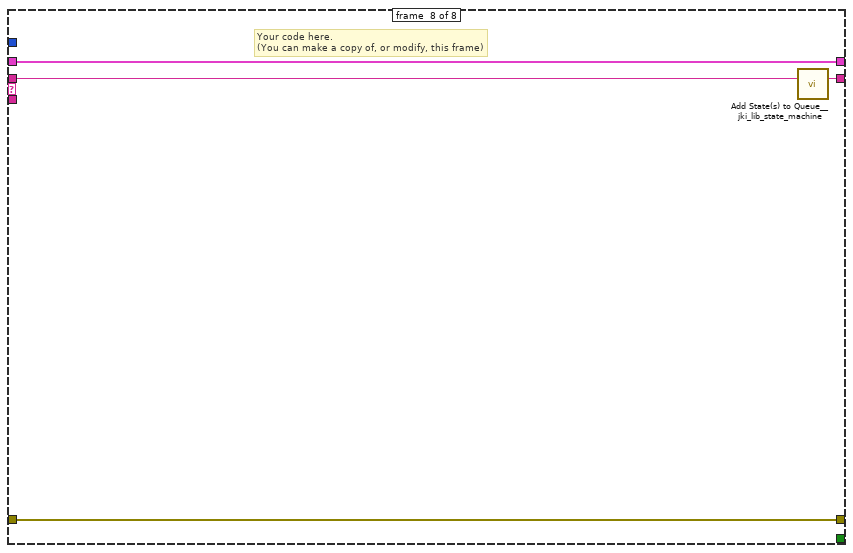
[diagram p12: hidden frame]
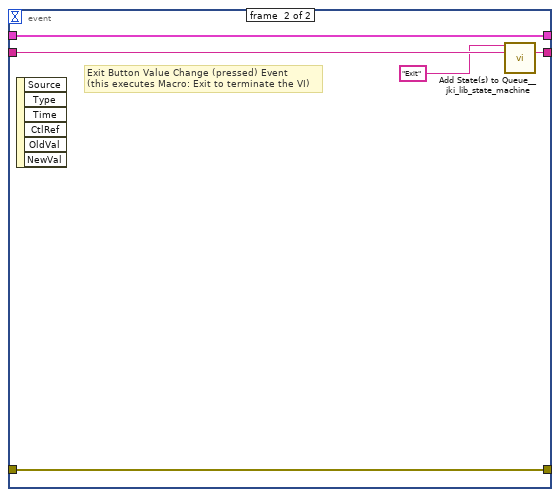
[diagram p13: hidden frame]
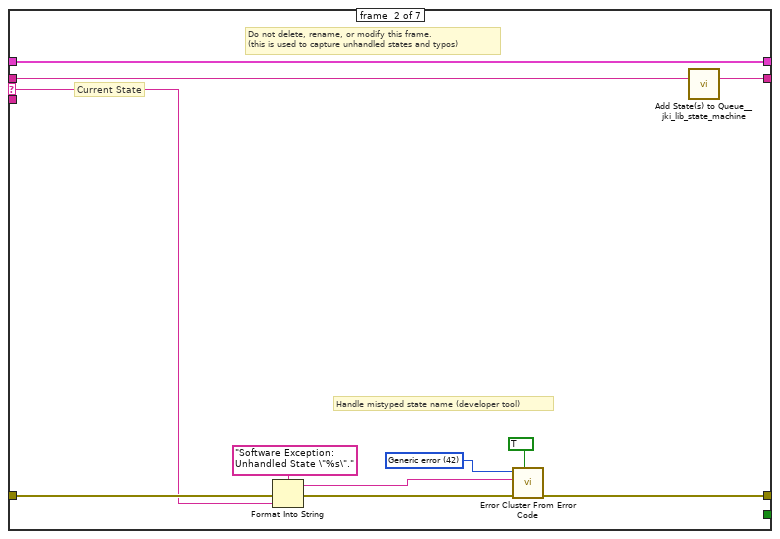
[diagram p14: hidden frame]
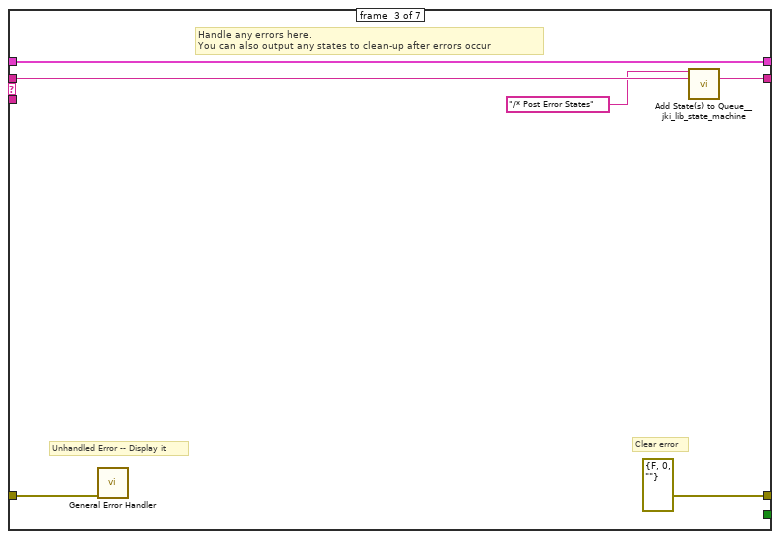
[diagram p15: hidden frame]
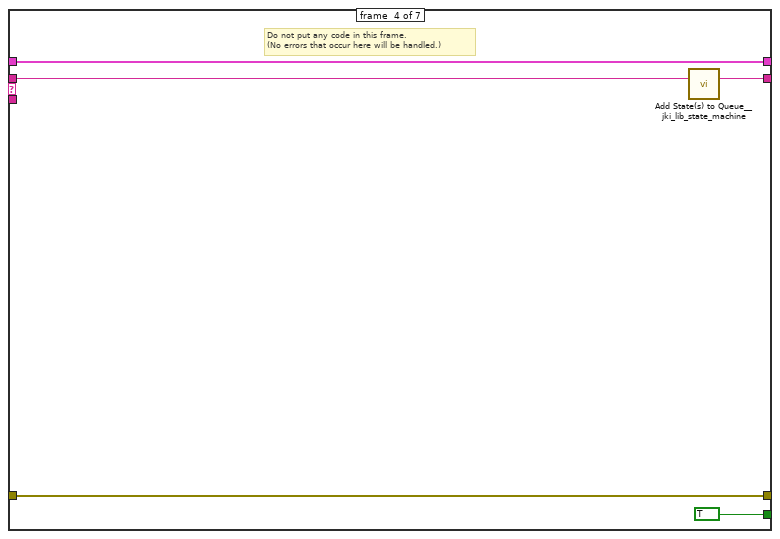
[diagram p16: hidden frame]
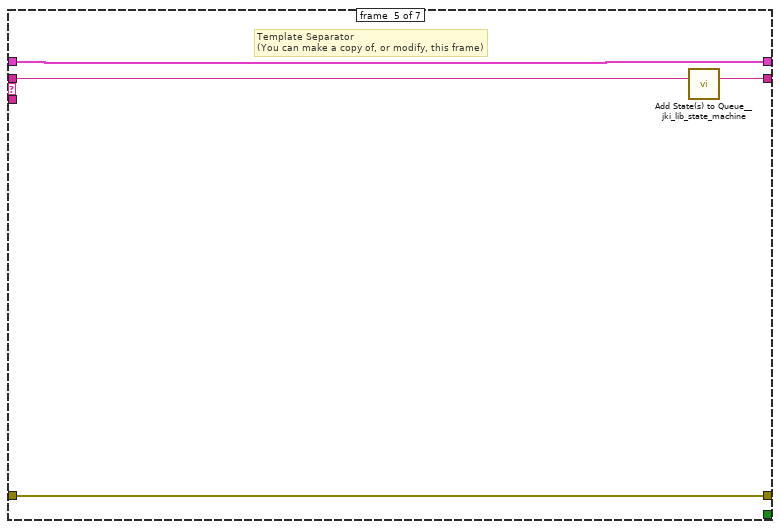
[diagram p17: hidden frame]
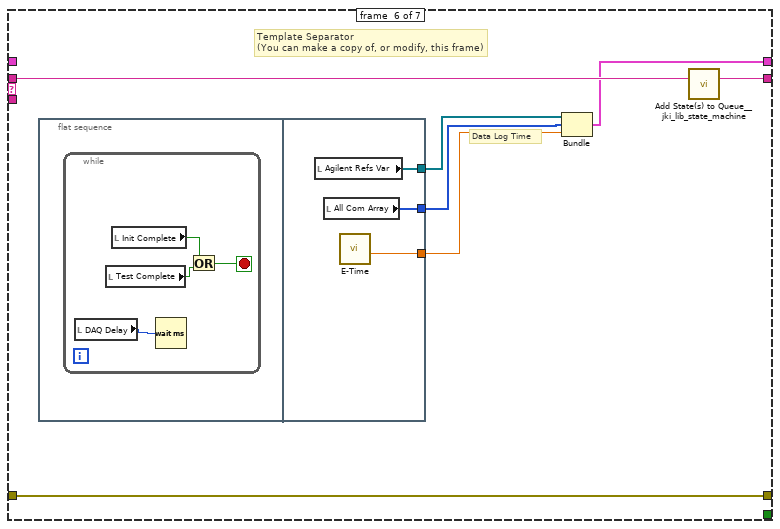
[diagram p18: hidden frame]
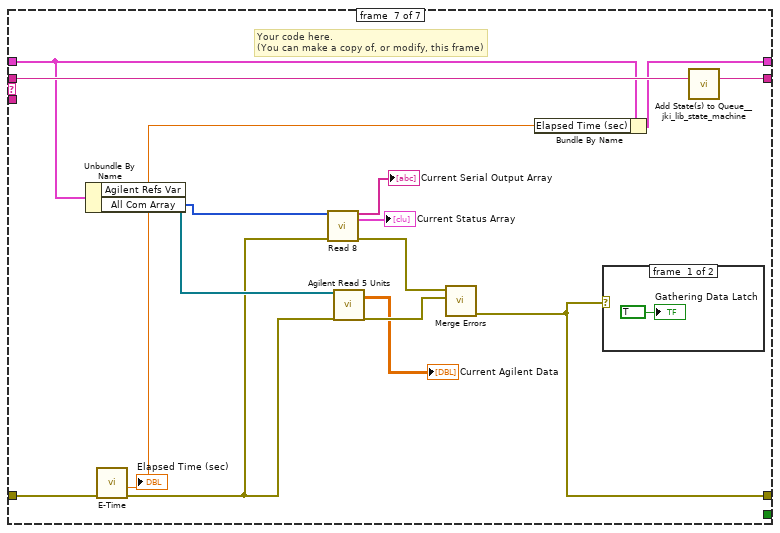
[diagram p19: hidden frame]
diagram:
  n1 = flat-sequence {
    tunnel: ["Macro: Initialize\nStart: DataLogging"] -> w7
    frame #0 {
      w11 = FALSE ("Init Complete")
      n2 = for {
        N: 56 -> [_]
        tunnel: [w16] -> w13 mode=indexing
        i -> [w20]
        n3 = Equal To 0?(x=w20) -> (x = 0?=w18:bool)
        n4 = Increment(x=w20) -> (x+1=w19:i32)
        n5 = Select(t=100, s=w18, f=w19) -> (s? t:f=w16:i32)
      }
      "All Com Array" <- w13
      n6 = local write "Elapsed Time (sec)"(0.0 ("Elapsed Time (sec)")) -> ()
      n7 = local write "Gathering Data Latch"(TRUE ("Gathering Data Latch")) -> ()
      n8 = local write "Init Complete"(w11) -> ()
      n9 = local write "Test Complete"(w11) -> ()
      n10 = local write "Stop Test"(w11) -> ()
      n11 = local write "DAQ Delay"(1000 ("DAQ Delay")) -> ()
    }
  }
  n12 = call <vilib>:"Add State(s) to Queue__jki_lib_state_machine.vi"("State(s) in (\"\")"=w7) -> ("States Out"=w8:string)  [unwired: 14 in]
  n13 = call <vilib>:"Add State(s) to Queue__jki_lib_state_machine.vi"("State(s) in (\"\")"="Data: Init") -> ("States Out"=w3:string)  [unwired: 14 in]
  n14 = call <vilib>:"Add State(s) to Queue__jki_lib_state_machine.vi"("State(s) in (\"\")"="Data: Init") -> ("States Out"=w6:string)  [unwired: 14 in]
  n15 = while "UI Loop" {
    shift-right: [w25] -> _
    shift-left: _ -> [w24]
    shift-right: [w27] -> _
    shift-left: _ -> [w22]
    shift-right: [w26] -> _
    shift-left: w8 -> [w28]
    tunnel: [w21] -> w1
    stop <- w21 stop-if-true
    w23 = -1  # Timeout
    n16 = call <vilib>:"Parse State Queue__jki_lib_state_machine.vi"("State Queue"=w28, "Error In (no error)"=w22) -> ("Remaining States"=w30:string, "Current State"=w31:string, "Arguments"=w29:string)  [unwired: 11 in]
    n17 = case shown="\"Agilent: Initialize\"" w31 {
      selector: w31 -> [_ _ w59 _ _ _ _ _ _ _ w217 _ _ _ _ _ _ _ _ _ _ _ _]
      tunnel: w30 -> [w38 w58 w63 w81 w88 w94 w98 w110 w138 w188 w220 w240 w288 w292 w296 w302 w313 w339 w344 w354 w358 w363 w367]
      tunnel: w29 -> [_ _ _ _ _ _ _ _ _ _ _ _ _ _ _ w297 w307 _ _ _ _ _ _]
      tunnel: w24 -> [w36 w55 w61 w72 w85 w92 w95 _ w124 w174 w216 w238 w283 w289 w294 w300 w309 w336 w341 w351 w355 w360 w364]
      tunnel: [w35 w56 w65 w78 errorcluster {"status"=FALSE, "code"=0, "source"=""} ("error out") w91 w96 w107 w136 w186 w218 w236 w284 w290 w293 w298 w310 w337 w342 w352 w356 w361 w365] -> w27
      tunnel: w22 -> [w34 w56 w64 w78 w84 w91 w96 w107 w136 w186 w215 w237 w285 w290 w293 w299 w311 w337 w342 w352 w356 w361 w365]
      tunnel: [w37 w57 w62 w80 w87 w93 w97 w109 w137 w187 w219 w239 w287 w291 w295 w301 w312 w338 w343 w353 w357 w362 w366] -> w26
      tunnel: [_ _ _ _ _ TRUE _ _ _ _ _ _ _ _ _ _ _ _ _ _ _ _ _] -> w21
      tunnel: [w33 w55 w61 w79 w85 w92 w95 w108 w124 w174 w216 w238 w283 w289 w294 w300 w309 w336 w341 w351 w355 w360 w364] -> w25
      tunnel: w23 -> [w32 _ _ _ _ _ _ _ _ _ _ _ _ _ _ _ _ _ _ _ _ _ _]
      frame #0 {
        n18 = event shown="[1] \"Stop Test\": Value Change" {
          selector: _ -> [_ _ _]
          dyn-events: _ -> [_ _ _]
          timeout: w32 -> [_ _ _]
          tunnel: w38 -> [w42 w48 w54]
          tunnel: [w41 w47 w53] -> w37
          tunnel: w36 -> [w39 w45 w51]
          tunnel: [w40 w46 w52] -> w35
          tunnel: w34 -> [w40 w46 w52]
          tunnel: [w39 w45 w51] -> w33
          event #0 {
            n19 = event-data() -> ()  [unwired: 1 in, 1 out]
            n20 = call <vilib>:"Add State(s) to Queue__jki_lib_state_machine.vi"("State(s) in (\"\")"=w42) -> ("States Out"=w41:string)  [unwired: 14 in]
          }
          event #1 {
            # "Exit Button Value Change (pressed) Event\n(this executes Macro: Exit to terminate the VI)"
            n21 = event-data() -> ()  [unwired: 1 in, 1 out]
            n22 = property on="Stop Test" class="Bool (strict)"("Val(Sgnl)"="Stop Test") -> ()  [unwired: 2 in, 2 out]
            n23 = call <vilib>:"Add State(s) to Queue__jki_lib_state_machine.vi"("State(s) in Front (\"\")"="Exit", "State(s) in (\"\")"=w48) -> ("States Out"=w47:string)  [unwired: 13 in]
          }
          event #2 {
            # "Discard the event because we'll close the front panel ourselves in Macro: Exit"
            # "Close Panel button (pressed) Event\n(this executes Macro: Exit to terminate the VI)"
            n24 = event-data() -> ()  [unwired: 1 in, 1 out]
            n25 = event-data("Discard?"=TRUE) -> ()  [unwired: 1 in, 1 out]
            n26 = call <vilib>:"Add State(s) to Queue__jki_lib_state_machine.vi"("State(s) in Front (\"\")"="Exit", "State(s) in (\"\")"=w54) -> ("States Out"=w53:string)  [unwired: 13 in]
          }
        }
      }
      frame #1 {
        # "Do not put any code in this frame.\n(it is a separator no-op)"
        n27 = call <vilib>:"Add State(s) to Queue__jki_lib_state_machine.vi"("State(s) in (\"\")"=w58) -> ("States Out"=w57:string)  [unwired: 14 in]
      }
      frame #2 {
        w68 = 42 items=["No error", "Argument error", "Memory is full", "Out of zone", "End of file", "File already open", "Generic file I/O error", "File not found", "File permission error", "Disk is full", "Duplicate path", "Too many files open", "System feature not enabled", "Resource file not found", "Cannot add resource", "Resource not found", "Image not found", "Image memory error", "Pen does not exist", "Config type invalid", "Config token not found", "Config parse error", "Config memory error", "Bad external code format", "Bad external code offset", "External code not present", "Null window", "Destroy window error", "Null menu", "Print aborted", "Bad print record", "Print driver error", "Windows error during printing", "Memory error during printing", "Print dialog error", "Generic print error", "Invalid device refnum", "Device not found", "Device parameter error", "Device unit error", "Cannot open device", "Device call aborted", "Generic error", "Cancelled by user", "Object ID too low", "Object ID too high", "Object not in heap", "Unknown heap", "Unknown object (invalid DefProc)", "Unknown object (DefProc not in table)", "Message out of range", "Invalid (null) method", "Unknown message", "Manager call not supported", "Bad address", "Network operation in progress", "Network operation timed out", "Connection is busy", "Network attribute not supported", "Network error", "Address in use", "System out of memory", "Connection aborted", "Connection refused", "Not connected", "Already connected", "Connection closed", "Initialization error (interapplication manager)", "Bad occurrence", "Wait on unbound occurrence handler", "Occurrence queue overflow", "Datalog type conflict", "Unused", "Unrecognized type (interapplication manager)", "Memory corrupt", "Failed to make temporary DLL", "Old CIN version", "Drag socket not found", "Failed to load drop-object", "Failed to register OLE object", "Failed to release OLE object", "Format specifier type mismatch", "Unknown format specifier", "Too few format specifiers", "Too many format specifiers", "Scan failed", "Newer CIN version", "Error converting to variant", "Runtime menu error", "Password tampered", "Variant attribute not found", "Incompatible variant data type", "Event data is not available", "Event Store is not present", "Occurrence is not found", "Event Queue is not created", "Event info is not available", "Refnum passed is NULL", "Error retrieving Class GUID", "Error retrieving CoClass GUID", "Error retrieving TypeLib GUID.", "Bad built application magic bytes.", "Specific driver is different from the specific driver associated with the Logical Name.", "There is no session opened to the class driver.", "Max Error", "MAX - Error with config objects", "MAX - Error loading configuration", "MAX - Group not supported"]
        # "Current State"
        # "Do not delete, rename, or modify this frame.\n(this is used to capture unhandled states and typos)"
        # "Handle mistyped state name (developer tool)"
        n28 = Format Into String(format string="Software Exception: Unhandled State \"%s\"." ("message"), error in=w64, w59) -> (resulting string=w67:string, error out=w66:errorcluster)  [unwired: 1 in]
        n29 = call <vilib>:"Error Cluster From Error Code.vi"("show call chain? (False)"=TRUE, "error in (no error)"=w66, "error message (\"\")"=w67, "error code (0)"=w68) -> ("error out"=w65:errorcluster)  [unwired: 5 in]
        n30 = call <vilib>:"Add State(s) to Queue__jki_lib_state_machine.vi"("State(s) in (\"\")"=w63) -> ("States Out"=w62:string)  [unwired: 14 in]
      }
      frame #3 {
        # "Do not delete, rename, or modify this frame.\n(this is used to determine panel behavior on exit)"
        # "originally closed?"
        # "exe?"
        # "If panel starts closed or is an EXE, then close it when we exit"
        n31 = property class="VI"() -> ("Front Panel.Open"=w77:bool)  [unwired: 2 in, 2 out]
        n32 = property class="App"() -> ("App.Kind"=w76:T4)  [unwired: 2 in, 2 out]
        n33 = control-ref of="Current VI Reference"() -> (w70:refnum<vi>)
        n34 = Not(x=w77) -> (.not. x?=w74:bool)
        n35 = Equal?(x=w76, y=T4."Run Time System" ("Application:Kind")) -> (x = y?=w73:bool)
        n36 = Or(x=w74, y=w73) -> (x .or. y?=w71:bool)
        n37 = Bundle By Name(cluster=w72, "Core.Current VI Reference"=w70, "Core.Close Panel on Exit?"=w71) -> (w79:T7)
        n38 = call <vilib>:"Add State(s) to Queue__jki_lib_state_machine.vi"("State(s) in (\"\")"=w81) -> ("States Out"=w80:string)  [unwired: 14 in]
      }
      frame #4 {
        # "Handle any errors here.\nYou can also output any states to clean-up after errors occur"
        # "Clear error"
        n39 = case shown="False" "Simulation" {
          tunnel: w84 -> [w89 _]
          frame #0 {
            # "Unhandled Error -- Display it"
            n40 = call <vilib>:"General Error Handler.vi"("error in (no error)"=w89) -> ()  [unwired: 10 in, 5 out]
          }
          frame #1 {
          }
        }
        n41 = call <vilib>:"Add State(s) to Queue__jki_lib_state_machine.vi"("State(s) in Front (\"\")"="/* Post Error States", "State(s) in (\"\")"=w88) -> ("States Out"=w87:string)  [unwired: 13 in]
      }
      frame #5 {
        # "Do not put any code in this frame.\n(No errors that occur here will be handled.)"
        n42 = call <vilib>:"Add State(s) to Queue__jki_lib_state_machine.vi"("State(s) in (\"\")"=w94) -> ("States Out"=w93:string)  [unwired: 14 in]
      }
      frame #6 {
        # "Do not put any code in this frame.\n(It is a separator no-op. You can make a copy of this frame to create a new Data frame)"
        n43 = call <vilib>:"Add State(s) to Queue__jki_lib_state_machine.vi"("State(s) in (\"\")"=w98) -> ("States Out"=w97:string)  [unwired: 14 in]
      }
      frame #7 {
        w104 = refnum<visa-resource-name>[] ["AGILENT1", "AGILENT2", "AGILENT3", "AGILENT4", "AGILENT5"]  # Agilent Refs
        w105 = refnum<vi>[] []  # UI Refs
        w106 = T8 {"Current VI Reference"=refnum, "Close Panel on Exit?"=FALSE}  # Core
        # "do not delete - used by framework"
        # "Data names and types of shift register data are defined by this bundle."
        # "Initialize the shift-register data, here.\n(data names are defined by what you wire into the bundle function)"
        n44 = global read "Globals Wilt.vi" "GUI Aisle 1A"() -> (w100:T2[])
        n45 = global read "Globals Wilt.vi" "GUI Aisle 4"() -> (w103:T2[])
        n46 = global read "Globals Wilt.vi" "GUI Aisle 3"() -> (w102:T2[])
        n47 = global read "Globals Wilt.vi" "GUI Aisle 2"() -> (w101:T2[])
        n48 = global read "Globals Wilt.vi" "GUI Aisle 1"() -> (w99:T2[])
        n49 = Bundle("Core"=w106, "UI Refs"=w105, "Agilent Refs"=w104, "GUI Aisle 4"=w103, "GUI Aisle 3"=w102, "GUI Aisle 2"=w101, "GUI Aisle 1A"=w100, "GUI Aisle 1"=w99) -> (w108:T7)  [unwired: 1 in]
        n50 = call <vilib>:"Add State(s) to Queue__jki_lib_state_machine.vi"("State(s) in (\"\")"=w110) -> ("States Out"=w109:string)  [unwired: 14 in]
        "Agilent Refs Var" <- w104
      }
      frame #8 {
        # "Initialization Macro\n(This is called once, when the VI starts)"
        n51 = for {
          N: 12 -> [_]
          tunnel: [w156] -> w127 mode=indexing
          i -> [w156]
        }
        n52 = for {
          N: 8 -> [_]
          tunnel: [w155] -> w130 mode=indexing
          i -> [w155]
        }
        n53 = Add(x=w127, y=45) -> (x+y=w126:i32[])
        n54 = Add(x=w127, y=21) -> (x+y=w120:i32[])
        n55 = Add(x=w127, y=33) -> (x+y=w121:i32[])
        n56 = Add(x=w130, y=13) -> (x+y=w116:i32[])
        n57 = Add(x=w127, y=1) -> (x+y=w117:i32[])
        n58 = global read "Globals Wilt.vi" "GUI Aisle 4"() -> (w125:T2[])
        n59 = global read "Globals Wilt.vi" "GUI Aisle 3"() -> (w123:T2[])
        n60 = global read "Globals Wilt.vi" "GUI Aisle 2"() -> (w122:T2[])
        n61 = global read "Globals Wilt.vi" "GUI Aisle 1A"() -> (w118:T2[])
        n62 = global read "Globals Wilt.vi" "GUI Aisle 1"() -> (w119:T2[])
        n63 = for {
          tunnel: w125 -> [w158] mode=indexing
          tunnel: w126 -> [w160] mode=indexing
          tunnel: [w157] -> w111 mode=indexing
          n64 = call "Update Wilt GUI.vi"("Dryer In"=w158, "Enum"=T5."Init Station Number", "Station Number In"=w160) -> ("Dryer Out"=w157:T2)  [unwired: 11 in, 1 out]
        }
        n65 = for {
          tunnel: w123 -> [w152] mode=indexing
          tunnel: w121 -> [w154] mode=indexing
          tunnel: [w151] -> w112 mode=indexing
          n66 = call "Update Wilt GUI.vi"("Dryer In"=w152, "Enum"=T5."Init Station Number", "Station Number In"=w154) -> ("Dryer Out"=w151:T2)  [unwired: 11 in, 1 out]
        }
        n67 = for {
          tunnel: w122 -> [w148] mode=indexing
          tunnel: w120 -> [w150] mode=indexing
          tunnel: [w147] -> w113 mode=indexing
          n68 = call "Update Wilt GUI.vi"("Dryer In"=w148, "Enum"=T5."Init Station Number", "Station Number In"=w150) -> ("Dryer Out"=w147:T2)  [unwired: 11 in, 1 out]
        }
        n69 = for {
          tunnel: w119 -> [w144] mode=indexing
          tunnel: w117 -> [w146] mode=indexing
          tunnel: [w143] -> w115 mode=indexing
          n70 = call "Update Wilt GUI.vi"("Dryer In"=w144, "Enum"=T5."Init Station Number", "Station Number In"=w146) -> ("Dryer Out"=w143:T2)  [unwired: 11 in, 1 out]
        }
        n71 = for {
          tunnel: w118 -> [w140] mode=indexing
          tunnel: w116 -> [w142] mode=indexing
          tunnel: [w139] -> w114 mode=indexing
          n72 = call "Update Wilt GUI.vi"("Dryer In"=w140, "Enum"=T5."Init Station Number", "Station Number In"=w142) -> ("Dryer Out"=w139:T2)  [unwired: 11 in, 1 out]
        }
        n73 = global write "Globals Wilt.vi" "GUI Aisle 4"(w111) -> ()
        n74 = global write "Globals Wilt.vi" "GUI Aisle 3"(w112) -> ()
        n75 = global write "Globals Wilt.vi" "GUI Aisle 2"(w113) -> ()
        n76 = global write "Globals Wilt.vi" "GUI Aisle 1A"(w114) -> ()
        n77 = global write "Globals Wilt.vi" "GUI Aisle 1"(w115) -> ()
        n78 = local write "GUI Aisle 3"(w112) -> ()
        n79 = local write "GUI Aisle 4"(w111) -> ()
        n80 = local write "GUI Aisle 2"(w113) -> ()
        n81 = local write "GUI Aisle 1A"(w114) -> ()
        n82 = local write "GUI Aisle 1"(w115) -> ()
        n83 = call <vilib>:"Add State(s) to Queue__jki_lib_state_machine.vi"("State(s) in (\"\")"=w138) -> ("States Out"=w137:string)  [unwired: 14 in]
      }
      frame #9 {
        # "Initialization Macro\n(This is called once, when the VI starts)"
        n84 = for {
          N: 12 -> [_]
          tunnel: [w206] -> w177 mode=indexing
          i -> [w206]
        }
        n85 = for {
          N: 8 -> [_]
          tunnel: [w205] -> w180 mode=indexing
          i -> [w205]
        }
        n86 = Add(x=w177, y=45) -> (x+y=w176:i32[])
        n87 = Add(x=w177, y=21) -> (x+y=w170:i32[])
        n88 = Add(x=w177, y=33) -> (x+y=w171:i32[])
        n89 = Add(x=w180, y=13) -> (x+y=w166:i32[])
        n90 = Add(x=w177, y=1) -> (x+y=w167:i32[])
        n91 = global read "Globals Wilt.vi" "GUI Aisle 4"() -> (w175:T2[])
        n92 = global read "Globals Wilt.vi" "GUI Aisle 3"() -> (w173:T2[])
        n93 = global read "Globals Wilt.vi" "GUI Aisle 2"() -> (w172:T2[])
        n94 = global read "Globals Wilt.vi" "GUI Aisle 1A"() -> (w168:T2[])
        n95 = global read "Globals Wilt.vi" "GUI Aisle 1"() -> (w169:T2[])
        n96 = for {
          tunnel: w175 -> [w208] mode=indexing
          tunnel: w176 -> [w210] mode=indexing
          tunnel: [w207] -> w161 mode=indexing
          n97 = call "Update Wilt GUI.vi"("Dryer In"=w208, "Enum"=T5."Init Station Number", "Station Number In"=w210) -> ("Dryer Out"=w207:T2)  [unwired: 11 in, 1 out]
        }
        n98 = for {
          tunnel: w173 -> [w202] mode=indexing
          tunnel: w171 -> [w204] mode=indexing
          tunnel: [w201] -> w162 mode=indexing
          n99 = call "Update Wilt GUI.vi"("Dryer In"=w202, "Enum"=T5."Init Station Number", "Station Number In"=w204) -> ("Dryer Out"=w201:T2)  [unwired: 11 in, 1 out]
        }
        n100 = for {
          tunnel: w172 -> [w198] mode=indexing
          tunnel: w170 -> [w200] mode=indexing
          tunnel: [w197] -> w163 mode=indexing
          n101 = call "Update Wilt GUI.vi"("Dryer In"=w198, "Enum"=T5."Init Station Number", "Station Number In"=w200) -> ("Dryer Out"=w197:T2)  [unwired: 11 in, 1 out]
        }
        n102 = for {
          tunnel: w169 -> [w194] mode=indexing
          tunnel: w167 -> [w196] mode=indexing
          tunnel: [w193] -> w165 mode=indexing
          n103 = call "Update Wilt GUI.vi"("Dryer In"=w194, "Enum"=T5."Init Station Number", "Station Number In"=w196) -> ("Dryer Out"=w193:T2)  [unwired: 11 in, 1 out]
        }
        n104 = for {
          tunnel: w168 -> [w190] mode=indexing
          tunnel: w166 -> [w192] mode=indexing
          tunnel: [w189] -> w164 mode=indexing
          n105 = call "Update Wilt GUI.vi"("Dryer In"=w190, "Enum"=T5."Init Station Number", "Station Number In"=w192) -> ("Dryer Out"=w189:T2)  [unwired: 11 in, 1 out]
        }
        n106 = global write "Globals Wilt.vi" "GUI Aisle 4"(w161) -> ()
        n107 = global write "Globals Wilt.vi" "GUI Aisle 3"(w162) -> ()
        n108 = global write "Globals Wilt.vi" "GUI Aisle 2"(w163) -> ()
        n109 = global write "Globals Wilt.vi" "GUI Aisle 1A"(w164) -> ()
        n110 = global write "Globals Wilt.vi" "GUI Aisle 1"(w165) -> ()
        n111 = local write "GUI Aisle 3"(w162) -> ()
        n112 = local write "GUI Aisle 4"(w161) -> ()
        n113 = local write "GUI Aisle 2"(w163) -> ()
        n114 = local write "GUI Aisle 1A"(w164) -> ()
        n115 = local write "GUI Aisle 1"(w165) -> ()
        n116 = call <vilib>:"Add State(s) to Queue__jki_lib_state_machine.vi"("State(s) in (\"\")"=w188) -> ("States Out"=w187:string)  [unwired: 14 in]
      }
      frame #10 {
        # "Do not put any code in this frame.\n(It is a separator no-op. You can make a copy of this frame to create a new Data frame)"
        n117 = Unbundle By Name(w216) -> ("Agilent Refs"=w212:refnum<visa-resource-name>[])
        "Agilent Refs" <- w212
        n118 = call "Agilent Channels.vi"() -> ("Station Data Headers"=→"Agilent Station Data Headers":string[][], "Index Array"=→"Agilent Station Data Index Array":i32[][], "Agilent Channels Array"=w211:T1[])  [unwired: 13 in]
        "Agilent Channels Array" <- w211
        n119 = for {
          tunnel: [w224] -> w218
          tunnel: w212 -> [w223] mode=indexing
          tunnel: w215 -> [w222]
          tunnel: w211 -> [w221]
          n120 = for {
            tunnel: w221 -> [w229] mode=indexing
            i -> [w228]
            n121 = Unbundle By Name(w229) -> ("Agilent Station"=w225:string)
            n122 = Increment(x=w228) -> (x+1=w227:i32)
            n123 = Number To Decimal String(width (-)=w227) -> (decimal integer string=w226:string)  [unwired: 1 in]
            n124 = Equal?(x=w225, y=w226) -> ()  [unwired: 1 out]
          }
          n125 = call "Init Agilent Channels Wilt.vi"("error in (no error)"=w222, "VISA Resource Name"=w223) -> ("error out"=w224:errorcluster)  [unwired: 17 in]
        }
        n126 = case shown="Error" w218 {
          selector: w218 -> [_ w232]
          tunnel: w217 -> [_ w233]
          frame #0 {
          }
          frame #1 {
            n127 = Unbundle By Name(w232) -> ("source"=w231:string)
            n128 = Concatenate Strings("Error: " ("string"), w233, w231) -> (w230:string)
            n129 = One Button Dialog(message=w230) -> ()  [unwired: 1 in, 1 out]
          }
        }
        n130 = call <vilib>:"Add State(s) to Queue__jki_lib_state_machine.vi"("State(s) in (\"\")"=w220) -> ("States Out"=w219:string)  [unwired: 14 in]
      }
      frame #11 {
        # "Do not put any code in this frame.\nInitialize all the com ports to GEA2 specs."
        n131 = local read "All Com Array"() -> (w235:i32[])
        n132 = while {
          shift-right: [w272] -> w236
          shift-left: w237 -> [w273]
          tunnel: w235 -> [w260]
          stop <- w259 stop-if-true
          w274 = T9."Init Com Port" ("Mode")
          n133 = Array Size(array=w260) -> (size(s)=w258:i32)
          n134 = Delete From Array(array=w260, length=8, index=0) -> (array with subset deleted=w249:i32[])  [unwired: 1 out]
          n135 = Index Array(array=w249, index #1=0 ("index"), index #2=1 ("index"), index #3=2 ("index"), index #4=3 ("index"), index #5=4 ("index"), index #6=5 ("index"), index #7=6 ("index"), index #8=7 ("index")) -> (element #1=w241:i32, element #2=w242:i32, element #3=w243:i32, element #4=w244:i32, element #5=w245:i32, element #6=w246:i32, element #7=w247:i32, element #8=w248:i32)
          n136 = call "Com Chan Type Conversion.vi"("Com Chan"=w243) -> ("VISA resource name"=w279:refnum<visa-resource-name>)  [unwired: 1 out]
          n137 = call "Com Chan Type Conversion.vi"("Com Chan"=w244) -> ("VISA resource name"=w280:refnum<visa-resource-name>)  [unwired: 1 out]
          n138 = call "Com Chan Type Conversion.vi"("Com Chan"=w241) -> ("VISA resource name"=w282:refnum<visa-resource-name>)  [unwired: 1 out]
          n139 = call "Com Chan Type Conversion.vi"("Com Chan"=w242) -> ("VISA resource name"=w281:refnum<visa-resource-name>)  [unwired: 1 out]
          n140 = call "Com Chan Type Conversion.vi"("Com Chan"=w247) -> ("VISA resource name"=w278:refnum<visa-resource-name>)  [unwired: 1 out]
          n141 = call "Com Chan Type Conversion.vi"("Com Chan"=w248) -> ("VISA resource name"=w277:refnum<visa-resource-name>)  [unwired: 1 out]
          n142 = call "Com Chan Type Conversion.vi"("Com Chan"=w245) -> ("VISA resource name"=w275:refnum<visa-resource-name>)  [unwired: 1 out]
          n143 = call "Com Chan Type Conversion.vi"("Com Chan"=w246) -> ("VISA resource name"=w276:refnum<visa-resource-name>)  [unwired: 1 out]
          n144 = call "GEA2_ICP_Dryer_SM.vi"("ComPort"=w279, "Mode"=w274) -> ("Error Out"=w269:errorcluster)  [unwired: 9 in, 4 out]
          n145 = call "GEA2_ICP_Dryer_SM.vi"("ComPort"=w280, "Mode"=w274, "Error In"=w273) -> ("Error Out"=w268:errorcluster)  [unwired: 8 in, 4 out]
          n146 = call "GEA2_ICP_Dryer_SM.vi"("ComPort"=w282, "Mode"=w274, "Error In"=w273) -> ("Error Out"=w271:errorcluster)  [unwired: 8 in, 4 out]
          n147 = call "GEA2_ICP_Dryer_SM.vi"("ComPort"=w281, "Mode"=w274, "Error In"=w273) -> ("Error Out"=w270:errorcluster)  [unwired: 8 in, 4 out]
          n148 = call "GEA2_ICP_Dryer_SM.vi"("ComPort"=w278, "Mode"=w274, "Error In"=w273) -> ("Error Out"=w265:errorcluster)  [unwired: 8 in, 4 out]
          n149 = call "GEA2_ICP_Dryer_SM.vi"("ComPort"=w277, "Mode"=w274, "Error In"=w273) -> ("Error Out"=w264:errorcluster)  [unwired: 8 in, 4 out]
          n150 = call "GEA2_ICP_Dryer_SM.vi"("ComPort"=w275, "Mode"=w274, "Error In"=w273) -> ("Error Out"=w267:errorcluster)  [unwired: 8 in, 4 out]
          n151 = call "GEA2_ICP_Dryer_SM.vi"("ComPort"=w276, "Mode"=w274, "Error In"=w273) -> ("Error Out"=w266:errorcluster)  [unwired: 8 in, 4 out]
          n152 = Build Array(w271, w270, w269, w268, w267, w266, w265, w264) -> (w263:errorcluster[])
          n153 = Greater Than 0?(x=w258) -> (x > 0?=w259:bool)
          n154 = call <vilib>:"Merge Errors.vi"("error array in"=w263) -> ("error out"=w272:errorcluster)  [unwired: 6 in]
        }
        n155 = call <vilib>:"Add State(s) to Queue__jki_lib_state_machine.vi"("State(s) in (\"\")"=w240) -> ("States Out"=w239:string)  [unwired: 14 in]
      }
      frame #12 {
        # "Cleanup any data and references, here.\n(this is called automatically, by the Macro: Exit)"
        n156 = Unbundle By Name(w283) -> ("Core.Current VI Reference"=w286:refnum<vi>)
        n157 = Close Reference(reference=w286, error in (no error)=w285) -> (error out=w284:errorcluster)
        n158 = call <vilib>:"Add State(s) to Queue__jki_lib_state_machine.vi"("State(s) in (\"\")"=w288) -> ("States Out"=w287:string)  [unwired: 14 in]
      }
      frame #13 {
        # "Do not put any code in this frame.\n(It is a separator no-op. You can make a copy of this frame to create a new UI frame)"
        n159 = call <vilib>:"Add State(s) to Queue__jki_lib_state_machine.vi"("State(s) in (\"\")"=w292) -> ("States Out"=w291:string)  [unwired: 14 in]
      }
      frame #14 {
        # "Initialize the User Interface, here.\n(this is called automatically, by the Macro: Init)"
        n160 = call <vilib>:"Add State(s) to Queue__jki_lib_state_machine.vi"("State(s) in (\"\")"=w296) -> ("States Out"=w295:string)  [unwired: 14 in]
      }
      frame #15 {
        # "Argument"
        # "Set and Unset Cursor Busy.\n(Usage: \"UI: Cursor Set >> Busy|Idle\")"
        n161 = case shown="\"Idle\", Default" w297 {
          tunnel: w299 -> [w304 w306]
          tunnel: [w303 w305] -> w298
          frame #0 {
            n162 = call <vilib>:"Unset Busy.vi"("error in (no error)"=w304) -> ("error out"=w303:errorcluster)  [unwired: 10 in]
          }
          frame #1 {
            n163 = call <vilib>:"Set Busy.vi"("error in (no error)"=w306) -> ("error out"=w305:errorcluster)  [unwired: 9 in, 1 out]
          }
        }
        n164 = call <vilib>:"Add State(s) to Queue__jki_lib_state_machine.vi"("State(s) in (\"\")"=w302) -> ("States Out"=w301:string)  [unwired: 14 in]
      }
      frame #16 {
        # "Argument"
        # "Set Front Panel Open or Closed\n(Usage: \"UI: Front Panel State >> Open|Close\")"
        n165 = Unbundle By Name(w309) -> ("Core.Current VI Reference"=w308:refnum<vi>)
        n166 = case shown="\"Open\", Default" w307 {
          tunnel: w311 -> [w317 w330]
          tunnel: [w319 w331] -> w310
          tunnel: w308 -> [w318 w328]
          frame #0 {
            n167 = property class="VI"(reference=w318, error in=w317) -> (reference out=w315:refnum<vi>, error out=w316:errorcluster, "Front Panel.Open"=w314:bool)
            n168 = case shown="False" w314 {
              tunnel: [w322 w325] -> w319
              tunnel: w316 -> [w321 w325]
              tunnel: w315 -> [w320 _]
              frame #0 {
                n169 = invoke class="VI" method="FP.Open"(reference=w320, error in=w321, "Activate"=TRUE, "State"=T6."Standard") -> (error out=w322:errorcluster)  [unwired: 1 in, 4 out]
              }
              frame #1 {
              }
            }
          }
          frame #1 {
            n170 = property class="VI"(reference=w328, error in=w330) -> (reference out=w327:refnum<vi>, error out=w329:errorcluster, "Front Panel.Open"=w326:bool)
            n171 = case shown="True" w326 {
              tunnel: [w332 w335] -> w331
              tunnel: w329 -> [w332 w334]
              tunnel: w327 -> [_ w333]
              frame #0 {
              }
              frame #1 {
                n172 = invoke class="VI" method="FP.Close"(reference=w333, error in=w334) -> (error out=w335:errorcluster)  [unwired: 1 in, 2 out]
              }
            }
          }
        }
        n173 = call <vilib>:"Add State(s) to Queue__jki_lib_state_machine.vi"("State(s) in (\"\")"=w313) -> ("States Out"=w312:string)  [unwired: 14 in]
      }
      frame #17 {
        # "Do not put any code in this frame.\n(It is a separator no-op. You can make a copy of this frame to create a new Macro frame)"
        n174 = call <vilib>:"Add State(s) to Queue__jki_lib_state_machine.vi"("State(s) in (\"\")"=w339) -> ("States Out"=w338:string)  [unwired: 14 in]
      }
      frame #18 {
        w340 = "Data: Initialize\nInitialize Core Data\nUI: Initialize\nUI: Front Panel State >> Open\nInit: Station Labels\nInit: Serial Numbers\nAgilent: Initialize\nCom: Initialize"  # Data: Initialize Initialize Core Data UI: Initialize UI: Front Panel State >> Open Init: Station Labels Init: Serial Numbers Agilent: Initialize Com: Initialize
        # "Initialization Macro\n(This is called once, when the VI starts)"
        n175 = call <vilib>:"Add State(s) to Queue__jki_lib_state_machine.vi"("State(s) in Front (\"\")"=w340, "State(s) in (\"\")"=w344) -> ("States Out"=w343:string)  [unwired: 13 in]
      }
      frame #19 {
        # "Exit Macro\n(This is called once, when the VI exits)"
        n176 = Unbundle By Name(w351) -> ("Core.Close Panel on Exit?"=w350:bool)
        n177 = Select(t="UI: Front Panel State >> Close", s=w350, f="") -> (s? t:f=w347:string)
        n178 = call <vilib>:"Add State(s) to Queue__jki_lib_state_machine.vi"("State(s) in (\"\")"=w347, "State(s) at Back (\"\")"="Data: Cleanup\nExit") -> ("States Out"=w345:string)  [unwired: 13 in]
        n179 = call <vilib>:"Add State(s) to Queue__jki_lib_state_machine.vi"("State(s) in Front (\"\")"=w345, "State(s) in (\"\")"=w354) -> ("States Out"=w353:string)  [unwired: 13 in]
      }
      frame #20 {
        # "Template Separator\n(You can make a copy of, or modify, this frame)"
        n180 = call <vilib>:"Add State(s) to Queue__jki_lib_state_machine.vi"("State(s) in (\"\")"=w358) -> ("States Out"=w357:string)  [unwired: 14 in]
      }
      frame #21 {
        w359 = TRUE ("Init Complete")
        # "Your code here.\n(You can make a copy of, or modify, this frame)"
        n181 = property on="Init Complete" class="Bool (strict)"("Val(Sgnl)"=w359) -> ()  [unwired: 2 in, 2 out]
        n182 = call <vilib>:"Add State(s) to Queue__jki_lib_state_machine.vi"("State(s) in (\"\")"=w363) -> ("States Out"=w362:string)  [unwired: 14 in]
        "Init Complete" <- w359
      }
      frame #22 {
        # "Your code here.\n(You can make a copy of, or modify, this frame)"
        n183 = call <vilib>:"Add State(s) to Queue__jki_lib_state_machine.vi"("State(s) in (\"\")"=w367) -> ("States Out"=w366:string)  [unwired: 14 in]
      }
    }
  }
  "Test Complete" <- w1
  n184 = while "UI State Machine" {
    shift-right: [w371] -> _
    shift-left: _ -> [w370]
    shift-right: [w374] -> _
    shift-left: _ -> [w368]
    shift-right: [w373] -> _
    shift-left: w3 -> [w375]
    stop <- w372 stop-if-true
    w369 = -1  # Timeout
    n185 = call <vilib>:"Parse State Queue__jki_lib_state_machine.vi"("State Queue"=w375, "Error In (no error)"=w368) -> ("Remaining States"=w377:string, "Current State"=w378:string, "Arguments"=w376:string)  [unwired: 11 in]
    n186 = case shown="\"\", \"Idle\"" w378 {
      selector: w378 -> [_ w426 _ _ _ _ _ _]
      tunnel: w377 -> [w385 w430 w442 w447 w451 w461 w482 w486]
      tunnel: w376 -> [_ _ _ _ _ _ _ _]
      tunnel: w370 -> [w383 w428 w439 w445 w448 _ w476 w483]
      tunnel: [w382 w432 errorcluster {"status"=FALSE, "code"=0, "source"=""} ("error out") w444 w449 w459 w477 w484] -> w374
      tunnel: w368 -> [w381 w431 w438 w444 w449 w459 w479 w484]
      tunnel: [w384 w429 w441 w446 w450 w460 w481 w485] -> w373
      tunnel: [_ _ _ TRUE _ _ _ _] -> w372
      tunnel: [w380 w428 w439 w445 w448 w458 w476 w483] -> w371
      tunnel: w369 -> [w379 _ _ _ _ _ _ _]
      frame #0 {
        # "executes when the state queue is empty"
        n187 = event shown="[2] \"GUI Aisle 4\": Value Change" {
          selector: _ -> [_ _ _]
          dyn-events: _ -> [_ _ _]
          timeout: w379 -> [_ _ _]
          tunnel: w385 -> [w389 w394 w403]
          tunnel: [w388 w393 w402] -> w384
          tunnel: w383 -> [w386 w391 w397]
          tunnel: [w387 w392 w398] -> w382
          tunnel: w381 -> [w387 w392 w398]
          tunnel: [w386 w391 w396] -> w380
          event #0 {
            n188 = event-data() -> ()  [unwired: 1 in, 1 out]
            n189 = call <vilib>:"Add State(s) to Queue__jki_lib_state_machine.vi"("State(s) in (\"\")"=w389) -> ("States Out"=w388:string)  [unwired: 14 in]
          }
          event #1 {
            # "Exit Button Value Change (pressed) Event\n(this executes Macro: Exit to terminate the VI)"
            n190 = event-data() -> ()  [unwired: 1 in, 1 out]
            n191 = call <vilib>:"Add State(s) to Queue__jki_lib_state_machine.vi"("State(s) in Front (\"\")"="Exit", "State(s) in (\"\")"=w394) -> ("States Out"=w393:string)  [unwired: 13 in]
          }
          event #2 {
            n192 = event-data() -> ("NewVal"=w395:T2[])  [unwired: 1 in, 5 out]
            n193 = for {
              tunnel: w395 -> [w425] mode=indexing
              tunnel: [w421] -> w405
              i -> [w421]
              stop <- w422 stop-if-true
              n194 = Unbundle By Name(w425) -> ("Boolean"=w424:bool)
              n195 = Equal?(x=w424, y=FALSE) -> (x = y?=w422:bool)
            }
            n196 = Array Size(array=w395) -> (size(s)=w406:i32)
            n197 = Greater?(x=w406, y=w405) -> (0:w404:bool)
            n198 = case shown="True" w404 {
              tunnel: w405 -> [_ w420]
              tunnel: w395 -> [_ w419]
              tunnel: [FALSE ("FileInit") w414] -> w401
              tunnel: [_ w413] -> w400
              frame #0 {
              }
              frame #1 {
                n199 = Index Array(array=w419, index=w420) -> (element=w417:T2)
                n200 = Unbundle By Name(w417) -> ("Dryer Details"=w416:T3)
                n201 = call "Panel Dryer Wilt Details.vi"("Dryer Details In"=w416) -> ("Dryer Details Out"=w415:T3)  [unwired: 14 in]
                n202 = call "Update Wilt GUI.vi"("Dryer In"=w417, "Enum"=T5."Update Detail Data", "Dryer Details In"=w415) -> ("Dryer Out"=w413:T2, "FileInit"=w414:bool)  [unwired: 11 in]
              }
            }
            n203 = case shown="True" w401 {
              tunnel: w400 -> [_ w408]
              tunnel: [_ "Create Save File" ("State(s) in Front (\"\")")] -> w399
              tunnel: w397 -> [w407 w410]
              tunnel: [w407 w409] -> w396
              frame #0 {
              }
              frame #1 {
                n204 = Bundle By Name(cluster=w410, "Dryer To Save"=w408) -> (w409:T10)
              }
            }
            n205 = call <vilib>:"Add State(s) to Queue__jki_lib_state_machine.vi"("State(s) in Front (\"\")"=w399, "State(s) in (\"\")"=w403) -> ("States Out"=w402:string)  [unwired: 13 in]
          }
        }
      }
      frame #1 {
        w435 = 42 items=["No error", "Argument error", "Memory is full", "Out of zone", "End of file", "File already open", "Generic file I/O error", "File not found", "File permission error", "Disk is full", "Duplicate path", "Too many files open", "System feature not enabled", "Resource file not found", "Cannot add resource", "Resource not found", "Image not found", "Image memory error", "Pen does not exist", "Config type invalid", "Config token not found", "Config parse error", "Config memory error", "Bad external code format", "Bad external code offset", "External code not present", "Null window", "Destroy window error", "Null menu", "Print aborted", "Bad print record", "Print driver error", "Windows error during printing", "Memory error during printing", "Print dialog error", "Generic print error", "Invalid device refnum", "Device not found", "Device parameter error", "Device unit error", "Cannot open device", "Device call aborted", "Generic error", "Cancelled by user", "Object ID too low", "Object ID too high", "Object not in heap", "Unknown heap", "Unknown object (invalid DefProc)", "Unknown object (DefProc not in table)", "Message out of range", "Invalid (null) method", "Unknown message", "Manager call not supported", "Bad address", "Network operation in progress", "Network operation timed out", "Connection is busy", "Network attribute not supported", "Network error", "Address in use", "System out of memory", "Connection aborted", "Connection refused", "Not connected", "Already connected", "Connection closed", "Initialization error (interapplication manager)", "Bad occurrence", "Wait on unbound occurrence handler", "Occurrence queue overflow", "Datalog type conflict", "Unused", "Unrecognized type (interapplication manager)", "Memory corrupt", "Failed to make temporary DLL", "Old CIN version", "Drag socket not found", "Failed to load drop-object", "Failed to register OLE object", "Failed to release OLE object", "Format specifier type mismatch", "Unknown format specifier", "Too few format specifiers", "Too many format specifiers", "Scan failed", "Newer CIN version", "Error converting to variant", "Runtime menu error", "Password tampered", "Variant attribute not found", "Incompatible variant data type", "Event data is not available", "Event Store is not present", "Occurrence is not found", "Event Queue is not created", "Event info is not available", "Refnum passed is NULL", "Error retrieving Class GUID", "Error retrieving CoClass GUID", "Error retrieving TypeLib GUID.", "Bad built application magic bytes.", "Specific driver is different from the specific driver associated with the Logical Name.", "There is no session opened to the class driver.", "Max Error", "MAX - Error with config objects", "MAX - Error loading configuration", "MAX - Group not supported"]
        # "Current State"
        # "Do not delete, rename, or modify this frame.\n(this is used to capture unhandled states and typos)"
        # "Handle mistyped state name (developer tool)"
        n206 = Format Into String(format string="Software Exception: Unhandled State \"%s\"." ("message"), error in=w431, w426) -> (resulting string=w434:string, error out=w433:errorcluster)  [unwired: 1 in]
        n207 = call <vilib>:"Error Cluster From Error Code.vi"("show call chain? (False)"=TRUE, "error in (no error)"=w433, "error message (\"\")"=w434, "error code (0)"=w435) -> ("error out"=w432:errorcluster)  [unwired: 5 in]
        n208 = call <vilib>:"Add State(s) to Queue__jki_lib_state_machine.vi"("State(s) in (\"\")"=w430) -> ("States Out"=w429:string)  [unwired: 14 in]
      }
      frame #2 {
        # "Unhandled Error -- Display it"
        # "Handle any errors here.\nYou can also output any states to clean-up after errors occur"
        # "Clear error"
        n209 = call <vilib>:"General Error Handler.vi"("error in (no error)"=w438) -> ()  [unwired: 10 in, 5 out]
        n210 = call <vilib>:"Add State(s) to Queue__jki_lib_state_machine.vi"("State(s) in Front (\"\")"="/* Post Error States", "State(s) in (\"\")"=w442) -> ("States Out"=w441:string)  [unwired: 13 in]
      }
      frame #3 {
        # "Do not put any code in this frame.\n(No errors that occur here will be handled.)"
        n211 = call <vilib>:"Add State(s) to Queue__jki_lib_state_machine.vi"("State(s) in (\"\")"=w447) -> ("States Out"=w446:string)  [unwired: 14 in]
      }
      frame #4 {
        # "Template Separator\n(You can make a copy of, or modify, this frame)"
        n212 = call <vilib>:"Add State(s) to Queue__jki_lib_state_machine.vi"("State(s) in (\"\")"=w451) -> ("States Out"=w450:string)  [unwired: 14 in]
      }
      frame #5 {
        # "Template Separator\n(You can make a copy of, or modify, this frame)"
        n213 = flat-sequence {
          tunnel: [w474] -> w457
          tunnel: [w473] -> w456
          tunnel: [w472] -> w455
          tunnel: [w471] -> w454
          tunnel: [w470] -> w453
          tunnel: ["Dryer To Save"] -> w452
          frame #0 {
            n214 = while {
              stop <- w466 stop-if-true
              n215 = local read "Gathering Data Latch"() -> (w462:bool)
              n216 = local read "Init Complete"() -> (w463:bool)
              n217 = local read "Test Complete"() -> (w467:bool)
              n218 = To Unsigned Long Integer(number="DAQ Delay") -> (unsigned 32bit integer=w465:u32)
              n219 = Wait (ms)(milliseconds to wait=w465) -> ()  [unwired: 1 out]
              n220 = And(x=w462, y=w463) -> (x .and. y?=w464:bool)
              n221 = Or(x=w464, y=w467) -> (x .or. y?=w466:bool)
            }
          }
          frame #1 {
            n222 = global read "Globals Wilt.vi" "GUI Aisle 1A"() -> (w473:T2[])
            n223 = global read "Globals Wilt.vi" "GUI Aisle 3"() -> (w471:T2[])
            n224 = global read "Globals Wilt.vi" "GUI Aisle 2"() -> (w472:T2[])
            n225 = global read "Globals Wilt.vi" "GUI Aisle 4"() -> (w470:T2[])
            n226 = global read "Globals Wilt.vi" "GUI Aisle 1"() -> (w474:T2[])
          }
        }
        n227 = Bundle("GUI Aisle 1"=w457, "GUI Aisle 1A"=w456, "GUI Aisle 2"=w455, "GUI Aisle 3"=w454, "GUI Aisle 4"=w453, "Dryer To Save"=w452) -> (w458:T10)  [unwired: 1 in]
        n228 = call <vilib>:"Add State(s) to Queue__jki_lib_state_machine.vi"("State(s) in (\"\")"=w461) -> ("States Out"=w460:string)  [unwired: 14 in]
      }
      frame #6 {
        w480 = TRUE  # Init
        # "Template Separator\n(You can make a copy of, or modify, this frame)"
        n229 = Unbundle By Name(w476) -> ("Dryer To Save"=w475:T2)
        n230 = call "File Wilt.vi"("Dryer In"=w475, "Data File Directory"="Data File Directory", "Init"=w480, "error in (no error)"=w479) -> ("error out"=w477:errorcluster)  [unwired: 11 in]
        n231 = call <vilib>:"Add State(s) to Queue__jki_lib_state_machine.vi"("State(s) in (\"\")"=w482) -> ("States Out"=w481:string)  [unwired: 14 in]
      }
      frame #7 {
        # "Your code here.\n(You can make a copy of, or modify, this frame)"
        n232 = call <vilib>:"Add State(s) to Queue__jki_lib_state_machine.vi"("State(s) in (\"\")"=w486) -> ("States Out"=w485:string)  [unwired: 14 in]
      }
    }
  }
  n233 = while "Data Acquisition State Machine" {
    shift-right: [w489] -> _
    shift-left: _ -> [w488]
    shift-right: [w492] -> _
    shift-left: _ -> [w487]
    shift-right: [w491] -> _
    shift-left: w6 -> [w493]
    stop <- w490 stop-if-true
    n234 = call <vilib>:"Parse State Queue__jki_lib_state_machine.vi"("State Queue"=w493, "Error In (no error)"=w487) -> ("Remaining States"=w495:string, "Current State"=w496:string, "Arguments"=w494:string)  [unwired: 11 in]
    n235 = case shown="\"Read Data\"" w496 {
      selector: w496 -> [_ w517 _ _ _ _ _]
      tunnel: w495 -> [w506 w521 w533 w538 w542 w549 w571]
      tunnel: w494 -> [_ _ _ _ _ _ _]
      tunnel: w488 -> [w501 w519 w530 w536 w539 _ w560]
      tunnel: [w504 w523 errorcluster {"status"=FALSE, "code"=0, "source"=""} ("error out") w535 w540 w547 w557] -> w492
      tunnel: w487 -> [w503 w522 w529 w535 w540 w547 w562]
      tunnel: [w505 w520 w532 w537 w541 w548 w570] -> w491
      tunnel: [_ _ _ TRUE _ _ _] -> w490
      tunnel: [w502 w519 w530 w536 w539 w546 w559] -> w489
      frame #0 {
        n236 = Unbundle By Name(w501) -> ("Elapsed Time (sec)"=w500:dbl)
        n237 = local read "DAQ Delay"() -> (w498:i32)
        n238 = call "E-Time.vi"() -> ("Elapsed Time (sec)"=w499:dbl)  [unwired: 9 in, 2 out]
        n239 = call "Timeout Calc.vi"("Complete time"=w499, "Gather Data Period"=w498, "Start Time"=w500) -> ("Delay Time"=w497:i32)  [unwired: 8 in]
        n240 = event shown="[0] Timeout" {
          selector: _ -> [_ _]
          dyn-events: _ -> [_ _]
          timeout: w497 -> [_ _]
          tunnel: w506 -> [w511 w516]
          tunnel: [w510 w515] -> w505
          tunnel: w501 -> [w508 w513]
          tunnel: [w509 w514] -> w504
          tunnel: w503 -> [w509 w514]
          tunnel: [w508 w513] -> w502
          event #0 {
            n241 = event-data() -> ()  [unwired: 1 in, 1 out]
            n242 = call <vilib>:"Add State(s) to Queue__jki_lib_state_machine.vi"("State(s) in (\"\")"=w511, "State(s) at Back (\"\")"="Read Data") -> ("States Out"=w510:string)  [unwired: 13 in]
          }
          event #1 {
            # "Exit Button Value Change (pressed) Event\n(this executes Macro: Exit to terminate the VI)"
            n243 = event-data() -> ()  [unwired: 1 in, 6 out]
            n244 = call <vilib>:"Add State(s) to Queue__jki_lib_state_machine.vi"("State(s) in Front (\"\")"="Exit", "State(s) in (\"\")"=w516) -> ("States Out"=w515:string)  [unwired: 13 in]
          }
        }
      }
      frame #1 {
        w526 = 42 items=["No error", "Argument error", "Memory is full", "Out of zone", "End of file", "File already open", "Generic file I/O error", "File not found", "File permission error", "Disk is full", "Duplicate path", "Too many files open", "System feature not enabled", "Resource file not found", "Cannot add resource", "Resource not found", "Image not found", "Image memory error", "Pen does not exist", "Config type invalid", "Config token not found", "Config parse error", "Config memory error", "Bad external code format", "Bad external code offset", "External code not present", "Null window", "Destroy window error", "Null menu", "Print aborted", "Bad print record", "Print driver error", "Windows error during printing", "Memory error during printing", "Print dialog error", "Generic print error", "Invalid device refnum", "Device not found", "Device parameter error", "Device unit error", "Cannot open device", "Device call aborted", "Generic error", "Cancelled by user", "Object ID too low", "Object ID too high", "Object not in heap", "Unknown heap", "Unknown object (invalid DefProc)", "Unknown object (DefProc not in table)", "Message out of range", "Invalid (null) method", "Unknown message", "Manager call not supported", "Bad address", "Network operation in progress", "Network operation timed out", "Connection is busy", "Network attribute not supported", "Network error", "Address in use", "System out of memory", "Connection aborted", "Connection refused", "Not connected", "Already connected", "Connection closed", "Initialization error (interapplication manager)", "Bad occurrence", "Wait on unbound occurrence handler", "Occurrence queue overflow", "Datalog type conflict", "Unused", "Unrecognized type (interapplication manager)", "Memory corrupt", "Failed to make temporary DLL", "Old CIN version", "Drag socket not found", "Failed to load drop-object", "Failed to register OLE object", "Failed to release OLE object", "Format specifier type mismatch", "Unknown format specifier", "Too few format specifiers", "Too many format specifiers", "Scan failed", "Newer CIN version", "Error converting to variant", "Runtime menu error", "Password tampered", "Variant attribute not found", "Incompatible variant data type", "Event data is not available", "Event Store is not present", "Occurrence is not found", "Event Queue is not created", "Event info is not available", "Refnum passed is NULL", "Error retrieving Class GUID", "Error retrieving CoClass GUID", "Error retrieving TypeLib GUID.", "Bad built application magic bytes.", "Specific driver is different from the specific driver associated with the Logical Name.", "There is no session opened to the class driver.", "Max Error", "MAX - Error with config objects", "MAX - Error loading configuration", "MAX - Group not supported"]
        # "Current State"
        # "Do not delete, rename, or modify this frame.\n(this is used to capture unhandled states and typos)"
        # "Handle mistyped state name (developer tool)"
        n245 = Format Into String(format string="Software Exception: Unhandled State \"%s\"." ("message"), error in=w522, w517) -> (resulting string=w525:string, error out=w524:errorcluster)  [unwired: 1 in]
        n246 = call <vilib>:"Error Cluster From Error Code.vi"("show call chain? (False)"=TRUE, "error in (no error)"=w524, "error message (\"\")"=w525, "error code (0)"=w526) -> ("error out"=w523:errorcluster)  [unwired: 5 in]
        n247 = call <vilib>:"Add State(s) to Queue__jki_lib_state_machine.vi"("State(s) in (\"\")"=w521) -> ("States Out"=w520:string)  [unwired: 14 in]
      }
      frame #2 {
        # "Unhandled Error -- Display it"
        # "Handle any errors here.\nYou can also output any states to clean-up after errors occur"
        # "Clear error"
        n248 = call <vilib>:"General Error Handler.vi"("error in (no error)"=w529) -> ()  [unwired: 10 in, 5 out]
        n249 = call <vilib>:"Add State(s) to Queue__jki_lib_state_machine.vi"("State(s) in Front (\"\")"="/* Post Error States", "State(s) in (\"\")"=w533) -> ("States Out"=w532:string)  [unwired: 13 in]
      }
      frame #3 {
        # "Do not put any code in this frame.\n(No errors that occur here will be handled.)"
        n250 = call <vilib>:"Add State(s) to Queue__jki_lib_state_machine.vi"("State(s) in (\"\")"=w538) -> ("States Out"=w537:string)  [unwired: 14 in]
      }
      frame #4 {
        # "Template Separator\n(You can make a copy of, or modify, this frame)"
        n251 = call <vilib>:"Add State(s) to Queue__jki_lib_state_machine.vi"("State(s) in (\"\")"=w542) -> ("States Out"=w541:string)  [unwired: 14 in]
      }
      frame #5 {
        # "Data Log Time"
        # "Template Separator\n(You can make a copy of, or modify, this frame)"
        n252 = flat-sequence {
          tunnel: [w556] -> w545
          tunnel: [w555] -> w544
          tunnel: [w554] -> w543
          frame #0 {
            n253 = while {
              stop <- w551 stop-if-true
              n254 = local read "DAQ Delay"() -> (w550:i32)
              n255 = local read "Test Complete"() -> (w552:bool)
              n256 = local read "Init Complete"() -> (w553:bool)
              n257 = Wait (ms)(milliseconds to wait=w550) -> ()  [unwired: 1 out]
              n258 = Or(x=w553, y=w552) -> (x .or. y?=w551:bool)
            }
          }
          frame #1 {
            n259 = local read "Agilent Refs Var"() -> (w556:refnum<visa-resource-name>[])
            n260 = local read "All Com Array"() -> (w555:i32[])
            n261 = call "E-Time.vi"() -> ("Elapsed Time (sec)"=w554:dbl)  [unwired: 9 in, 2 out]
          }
        }
        n262 = Bundle("Agilent Refs Var"=w545, "All Com Array"=w544, "Elapsed Time (sec)"=w543) -> (w546:T11)  [unwired: 1 in]
        n263 = call <vilib>:"Add State(s) to Queue__jki_lib_state_machine.vi"("State(s) in (\"\")"=w549) -> ("States Out"=w548:string)  [unwired: 14 in]
      }
      frame #6 {
        # "Your code here.\n(You can make a copy of, or modify, this frame)"
        n264 = Unbundle By Name(w560) -> ("Agilent Refs Var"=w565:refnum<visa-resource-name>[], "All Com Array"=w564:i32[])
        n265 = call "E-Time.vi"("error in (no error)"=w562) -> ("error out"=w561:errorcluster, "Elapsed Time (sec)"=w558:dbl)  [unwired: 8 in, 1 out]
        "Elapsed Time (sec)" <- w558
        n266 = call "Read 8.vi"("Com Array"=w564, "error in (no error)"=w561) -> ("Output array"=→"Current Serial Output Array":string[], "Status Array"=→"Current Status Array":cluster{"Color":u32, "Status":string}[], "error out"=w569:errorcluster)  [unwired: 11 in]
        n267 = call "Agilent Read 5 Units.vi"("Agilent Refs"=w565, "error in (no error)"=w561) -> ("All Agilent Data"=→"Current Agilent Data":dbl[][], "error out"=w568:errorcluster)  [unwired: 16 in]
        n268 = call <vilib>:"Merge Errors.vi"("error in 2 (no error)"=w568, "error in 1 (no error)"=w569) -> ("error out"=w557:errorcluster)  [unwired: 5 in]
        n269 = Bundle By Name(cluster=w560, "Elapsed Time (sec)"=w558) -> (w559:T11)
        n270 = case shown="No Error" w557 {
          frame #0 {
            "Gathering Data Latch" <- TRUE
          }
          frame #1 {
          }
        }
        n271 = call <vilib>:"Add State(s) to Queue__jki_lib_state_machine.vi"("State(s) in (\"\")"=w571) -> ("States Out"=w570:string)  [unwired: 14 in]
      }
    }
  }
  n272 = Not(x=w1) -> (.not. x?=w2:bool)
  n273 = property on="Test Complete" class="Bool (strict)"("Val(Sgnl)"=w1) -> ()  [unwired: 2 in, 2 out]
  n274 = local write "Stop Test"(w2) -> ()
